vi "Micro-PL v10.6.1.vi"() -> ()   [LabVIEW 2010]
uses:
  drivers/Oxford ITC/ITCAPPS.LLB/ITCSetup.ctl
  drivers/Oxford ITC/ITCSUBS.LLB/ITCIO.ctl
  drivers/Oxford ITC/BUSGEN.LLB/OxfordAddress.ctl
  drivers/Oxford ITC/ITCSUBS.LLB/ITCVersion.ctl
  subvi/NPC3SG/TypeDefs/NPC3SG Live Controls.ctl
  subvi/NPC3SG/TypeDefs/NPC3SG Current Values.ctl
  subvi/NPC3SG/TypeDefs/NPC3SG Set Positions.ctl
  subvi/ITC503/TypeDefs/ITC503 Settings.ctl
  subvi/ITC503/TypeDefs/ITC503 Current Values.ctl
  subvi/iHR550/TypeDefs/iHR Current Values.ctl
  subvi/iHR550/TypeDefs/iHR Settings.ctl
  subvi/Mapping/TypeDefs/Mapping Spectra Params.ctl
  <vilib>/Utility/miscctls.llb/LVBoundsTypeDef.ctl
  subvi/Symphony/TypeDefs/Symphony Area Format.ctl
  <vilib>/Utility/miscctls.llb/LVPointTypeDef.ctl
  subvi/Mapping/TypeDefs/Mapping Input Parameters v10.6.0.ctl
  subvi/Global Variables.vi
  <vilib>/Analysis/NI_AALBase.lvlib
panel:
  out "Spectrum Raw PX":dbl[][](array[numeric])
  out "Image Raw":i32[][](array[numeric])
  in  "Wavelength Recalculate":bool
  out "CCD Error":errorcluster
  out "Firmware":string="V1.20 CCD_4000"
  out "CCD Gain Number":i32[](array[numeric])=[10, 11, 12, 13, 8, 2]
  out "CCD ADC Number":i32[](array[numeric])=[0, 1, 2, 3, 4]
  out "JYCCDLib.IJYCCDReqd":refnum<k7>
  out "Spectrum Raw WL":dbl[][](array[numeric])
  out "Mapping State Storage":bool
  out "Drive Copy Target":bool
  in  "CCD Shutter":bool caption="Shutter:"
  out "Measurement Running":bool
  out "ITC Running":bool
  out "Drive Running":bool
  out "CCD Running":bool
  out "Mono Running":bool
  in  "Exit":bool
  out "Mono Status":bool
  out "Drive Status":bool
  out "CCD Status":bool
  out "ITC Status":bool
  in  "Register":enum32{"Devices", "Acquisition / Mapping"}(tab)
  out "CCD Temp Graph":dbl(graph)=-134.538067
  in  "CCD Gain":u16(ring)=1 caption="Gain Mode" items=["High Light", "Best Dynamic Range", "High Sensitivity"]
  in  "Image Mode":bool caption="Image Mode?"
  in  "CCD Names":u16(ring) caption="CCD ID" items=["Symphony II"]
  in  "CCD Connect":bool
  out "CCD Temperature":dbl caption="Temp. (K)" min=10.0 max=160.0 step=0.1 format="%.1f"
  out "CCD Pixel X":i32=2048 caption="X Pixels"
  out "CCD Pixel Y":i32=512 caption="Y Pixels"
  out "CCD Data Size":i32=2048 caption="Data Size"
  in  "CCD ADC":u16(ring) caption="ADC Frequency" items=["20 kHz       ", " 1 MHz       ", " 1 MHz Ultra ", "500 kHz Wrap"]
  in  "CCD Configure":bool
  in  "CCD Area":T1={"XStart"=1, "YStart"=1, "XStop"=2048, "YStop"=512, "XBin"=1, "YBin"=1}
  in  "Snapshot Folder":path=path "C:/Users/WET-KORR/Desktop/Screenshots"
  in  "Camera Name":string="HD USB Camera"
  out "CCD IDs":u16(ring) items=["CCD1"]
  out "ITC Current Values":T2 {"ITC503 Gradient" format="%.2f"; "ITC503 Setpoint" min=-273.0 max=300000.0 step=0.0001 format="%.1f"; "ITC503 I" format="%_1f"; "ITC503 P" format="%_1f"; "ITC503 Temperature" min=0.0 max=1645.0 step=1e-05 format="%.2f"; "ITC503 Heater" min=0.0 max=100.0 step=0.01 scale=0.0..100.0}
  in  "ITC Settings":T3={"ITC503 Set Setpoint"=0.0, "ITC503 Set Auto Heater"=TRUE, "ITC503 Set Auto PID"=TRUE, "P"=0.0, "I"=0.0, "D"=0.0} {"D" min=0.0 max=100.0 step=0.1 format="%.1f"; "I" min=0.0 max=100.0 step=0.1 format="%.1f"; "P" min=0.0 max=100.0 step=0.1 format="%.1f"; "ITC503 Set Setpoint" min=-273.0 max=300000.0 step=0.1 format="%.1f"}
  in  "ITC Configure":bool
  in  "ITC Connect":bool
  in  "ITC Selector":u16(ring) caption="Select Device" items=["ITC503s"]
  out "Drive Current Values":T4 {"Drive Z Position" min=-273.0 max=300000.0 step=0.0001 format="%.3f"; "Drive Y Position" min=-273.0 max=300000.0 step=0.0001 format="%.3f"; "Drive X Position" min=-273.0 max=300000.0 step=0.0001 format="%.3f"}
  in  "Drive Connection":refnum<visa-resource-name>="COM6" caption="COM Port"
  in  "Drive Connect":bool
  in  "Mono Force Init":bool=TRUE caption="iHR550 Force Init"
  in  "Mono Connect":bool
  in  "Mono ID":string(combo)="iHR550" caption="Monochromator ID"
  out "Mono Timing":u32 caption="Mono"
  out "Drive Timing":u32 caption="Drive"
  out "ITC Timing":u32 caption="ITC"
  out "CCD Timing":u32 caption="CCD"
  in  "Spectrum Axis":u16(ring)=1 caption="Axis" items=["Pixel", "Wavelength", "Energy"]
  in  "Spectrum Autosave":bool caption="iHR550 Force Init"
  in  "CCD Preview":bool
  in  "CCD Acquire":bool
  in  "Spectrum Settings":T5={"Integration Time"=1.0, "Repetitions"=1, "Mapping Spectra"=TRUE} caption="Mapping Spectra Settings" {"Repetitions" min=1 max=100 step=1; "Integration Time" min=0.1 max=6000.0 step=0.1 format="%.1f"}
  in  "CCD Current Rep.":string="0/0"
  out "Spectrum":cluster{dbl[], dbl[]}[](graph)
  in  "Spectrum Noise":i64 caption="Noise Level"
  in  "Spectrum Load":bool
  in  "Spectrum Save":bool
  out "Image":dbl[][](graph)
  in  "Spectrum Maximize":bool
  in  "Video Show":bool
  in  "Drive GoTo":bool caption="Objective Move Abs."
  in  "Drive New Positions":T6 {"Drive X Set" min=10.0 max=160.0 step=0.1 format="%.3f"; "Drive Z Set" min=10.0 max=160.0 step=0.1 format="%.3f"; "Drive Y Set" min=10.0 max=160.0 step=0.1 format="%.3f"}
  out "Drive Live Current Values":T4 {"Drive Z Position" min=-273.0 max=300000.0 step=0.0001 format="%.3f"; "Drive Y Position" min=-273.0 max=300000.0 step=0.0001 format="%.3f"; "Drive X Position" min=-273.0 max=300000.0 step=0.0001 format="%.3f"}
  in  "Drive Live Controls":T7={"Snapshot"=FALSE, "Move Step"=0.5, "Move Home"=FALSE, "Move Down"=FALSE, "Move Up"=FALSE, "Move Left"=FALSE, "Move Right"=FALSE, "Move Out"=FALSE, "Move In"=FALSE} {"Move Step" min=0.0 max=30.0 step=0.1 format="%.3f"}
  in  "Mapping Start":bool
  in  "Mono Configure":bool
  in  "Mono Settings":T8={"iHR550 Set Exit Mirror"=2, "iHR550 Set Side Exit"=0.0, "iHR550 Set Front Entrance"=0.0, "iHR550 Set Wavelength"=897.9988, "iHR550 Set Grating"=0, "iHR550 Set Grating Switch"=FALSE, "iHR550 Set Wavelength Switch"=FALSE, "iHR550 Set Mirror Switch"=FALSE, "iHR550 Set Slits Switch"=FALSE} {"iHR550 Set Grating" items=["1800"=1, "600"=2, "150"=3]; "iHR550 Set Wavelength" min=0.0 max=1500.0 step=1.0; "iHR550 Set Side Exit" min=0.0 max=2000.0 step=1.0; "iHR550 Set Exit Mirror" items=["Front"=2, "Side"=3]}
  out "Mono Current Values":T9={"iHR 550 Front Entrance"=0.0, "iHR550 Side Exit"=0.0, "iHR550 Wavelength"=897.9988, "iHR550 Exit Mirror"=2, "iHR550 Grating"="1", "Grating Index"=1} {"iHR550 Exit Mirror" items=["EntranceMirror", "ExitMirror", "Front", "Side"]}
  out "ITC Temp Storage":dbl
  out "Runtime":u32
  out "ITC Gradient Time":i64
  out "ITC Read":bool
  out "CCD Read":bool
  out "Mono Read":bool
  out "Drive Read":bool
  out "Spectrum Properties":cluster{"Position":T10, "Plot Area Size":T10}={"Position"={"Width"=36, "Height"=367}, "Plot Area Size"={"Width"=496, "Height"=264}}
  in  "Auto Folder":path caption="Ausgewählter Pfad"
  out "Wavelengths (nm)":dbl[](array[numeric])
  out "iHR550 RefNum":refnum<k7> caption="Mono RefNum out"
  out "ITC Setup":T11={"Description"="", "IO Info"={"Address"={"Com Port"=1, "ISOBUS Address"=1, "GPIB Address"=24, "Communication"=enum."ISOBUS"}, "Version"=enum."ITC503", "Ch 1 dec places"=1, "Ch 2 dec places"=1, "Ch 3 dec places"=1, "Ch1 Name"="", "Ch2 Name"="", "Ch3 Name"=""}}
  # "Correlation Setup"
  # "Active"
  # "Active"
  # "ITC"
  # "iHR"
  # "Drive"
  # "CCD"
  # "Status"
  # "CCD"
  # "ITC"
  # "iHR"
  # "Drive"
  # "CCD"
  # "Video"
  # "Cryostat"
  # "Objective Drive"
  # "Monochromator"
  # "Timing"
  # "CCD"
  # "Acquisition"
  # "Drive Control"
  # "XY"
  # "Z"
  # "Mapping"
  # "Launch the Spectral Mapping VI and Raman Tool Set 2.0 in a new window."
  # "Monochromator"
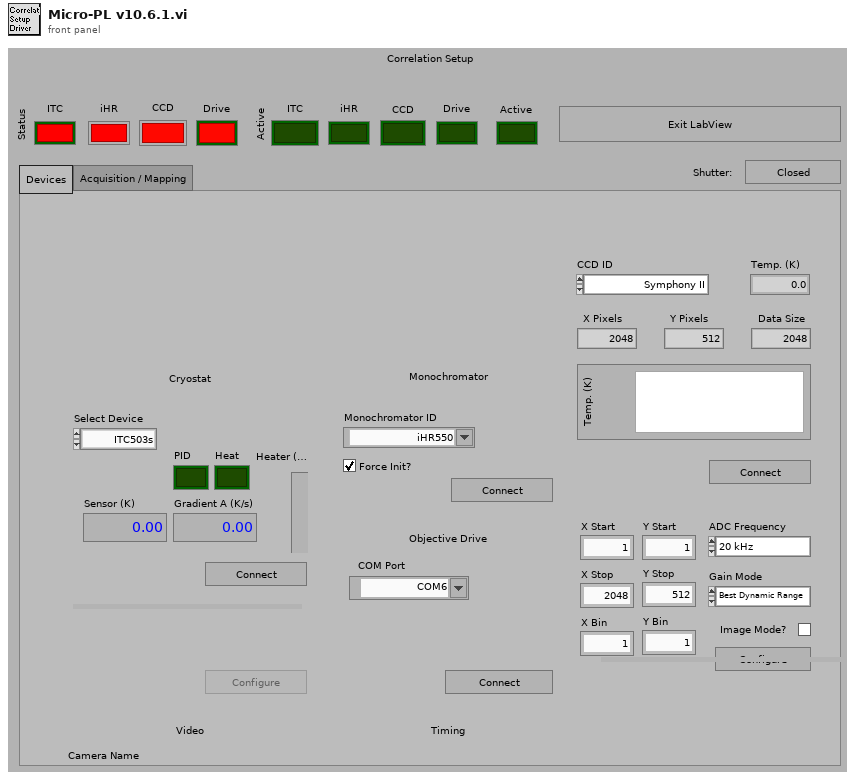
[diagram p1: front panel]
types:
  T1 = typedef "Symphony Area Format.ctl" = cluster{"XStart":i32, "YStart":i32, "XStop":i32, "YStop":i32, "XBin":i32, "YBin":i32}
  T2 = typedef "ITC503 Current Values.ctl" = cluster{"ITC503 Heater":dbl, "ITC503 Temperature":dbl, "ITC503 P":dbl, "ITC503 I":dbl, "ITC503 D":dbl, "ITC503 Setpoint":dbl, "ITC503 Gradient":dbl, "ITC503 Heater Auto":bool, "ITC503 PID Auto":bool}
  T3 = typedef "ITC503 Settings.ctl" = cluster{"ITC503 Set Setpoint":dbl, "ITC503 Set Auto Heater":bool, "ITC503 Set Auto PID":bool, "P":dbl, "I":dbl, "D":dbl}
  T4 = typedef "NPC3SG Current Values.ctl" = cluster{"Drive X Position":dbl, "Drive Y Position":dbl, "Drive Z Position":dbl}
  T5 = typedef "Mapping Spectra Params.ctl" = cluster{"Integration Time":dbl, "Repetitions":u16, "Mapping Spectra":bool}
  T6 = typedef "NPC3SG Set Positions.ctl" = cluster{"Drive X Set":dbl, "Drive Y Set":dbl, "Drive Z Set":dbl}
  T7 = typedef "NPC3SG Live Controls.ctl" = cluster{"Snapshot":bool, "Move Step":dbl, "Move Home":bool, "Move Down":bool, "Move Up":bool, "Move Left":bool, "Move Right":bool, "Move Out":bool, "Move In":bool}
  T8 = typedef "iHR Settings.ctl" = cluster{"iHR550 Set Exit Mirror":u16, "iHR550 Set Side Exit":dbl, "iHR550 Set Front Entrance":dbl, "iHR550 Set Wavelength":dbl, "iHR550 Set Grating":u16, "iHR550 Set Grating Switch":bool, "iHR550 Set Wavelength Switch":bool, "iHR550 Set Mirror Switch":bool, "iHR550 Set Slits Switch":bool}
  T9 = typedef "iHR Current Values.ctl" = cluster{"iHR 550 Front Entrance":dbl, "iHR550 Side Exit":dbl, "iHR550 Wavelength":dbl, "iHR550 Exit Mirror":i32, "iHR550 Grating":string, "Grating Index":i32}
  T10 = typedef "LVBoundsTypeDef.ctl" = cluster{"Width":u32, "Height":u32}
  T11 = typedef "ITCSetup.ctl" = cluster{"Description":string, "IO Info":T12}
  T12 = typedef "ITCIO.ctl" = cluster{"Address":T13, "Version":T14, "Ch 1 dec places":i16, "Ch 2 dec places":i16, "Ch 3 dec places":i16, "Ch1 Name":string, "Ch2 Name":string, "Ch3 Name":string}
  T13 = typedef "OxfordAddress.ctl" = cluster{"Com Port":i32, "ISOBUS Address":i32, "GPIB Address":i16, "Communication":enum16{"RS232", "ISOBUS", "GPIB", "Gateway"}}
  T14 = typedef "ITCVersion.ctl" = enum16{"ITC502", "ITC503", "ITC601"}
  T15 = enum8{"Enabled", "Disabled", "Disabled and Grayed Out"}
  T16 = typedef "LVPointTypeDef.ctl" = cluster{"Horizontal":i16, "Vertical":i16}
  T17 = enum16{"fire", "rainbow", "gray", "inverse gray", "ice", "original"}
  T18 = typedef "Mapping Input Parameters v10.6.0.ctl" = cluster{"Drive Connection Port":refnum<visa-resource-name>, "ITC503 Current Values":T2, "Wavelengths (nm)":dbl[], "Drive Current Values":T4, "iHR Current Values":T9, "Spectra Settings":T5, "CCD3500 Temperature":dbl, "Simulate Drive":bool, "Simulate Spectra":bool, "JYCCDLib.IJYCCDReqd":refnum<k7>, "CCD Area":T1, "CCD Gain":u16, "CCD ADC":u16}
  T19 = cluster{"Intensities":dbl[], "Wavelengths":dbl[]}[]
  T20 = typedef "LVPositionTypeDef.ctl" = cluster{"Left":i32, "Top":i32}
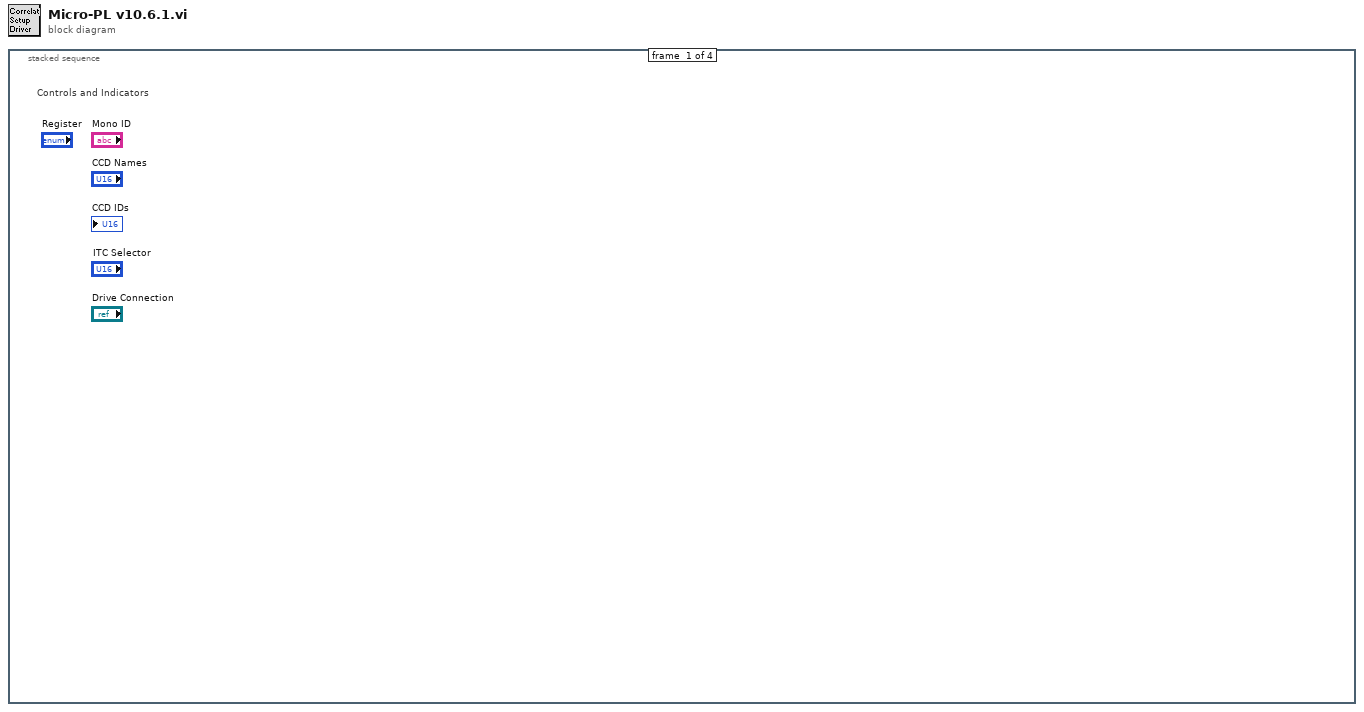
[diagram p0: block diagram]
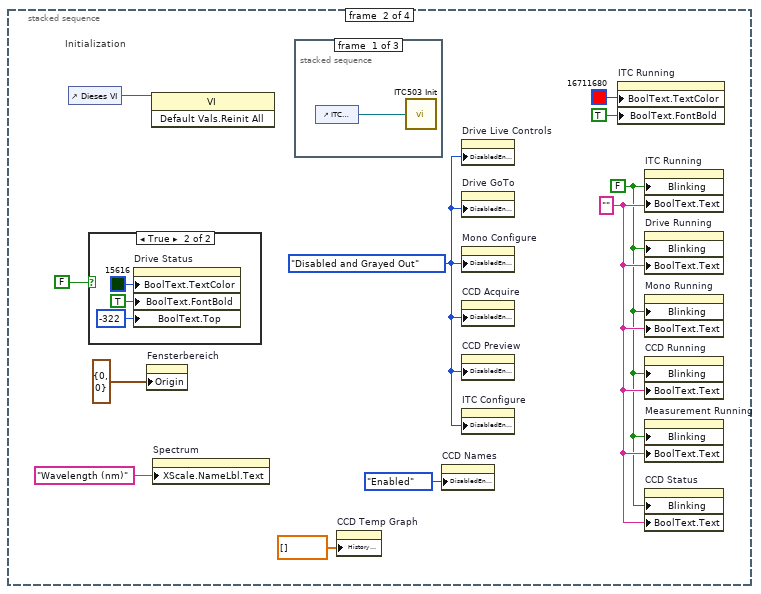
[diagram p2: hidden frame]
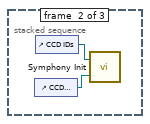
[diagram p3: hidden frame]
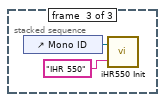
[diagram p4: hidden frame]
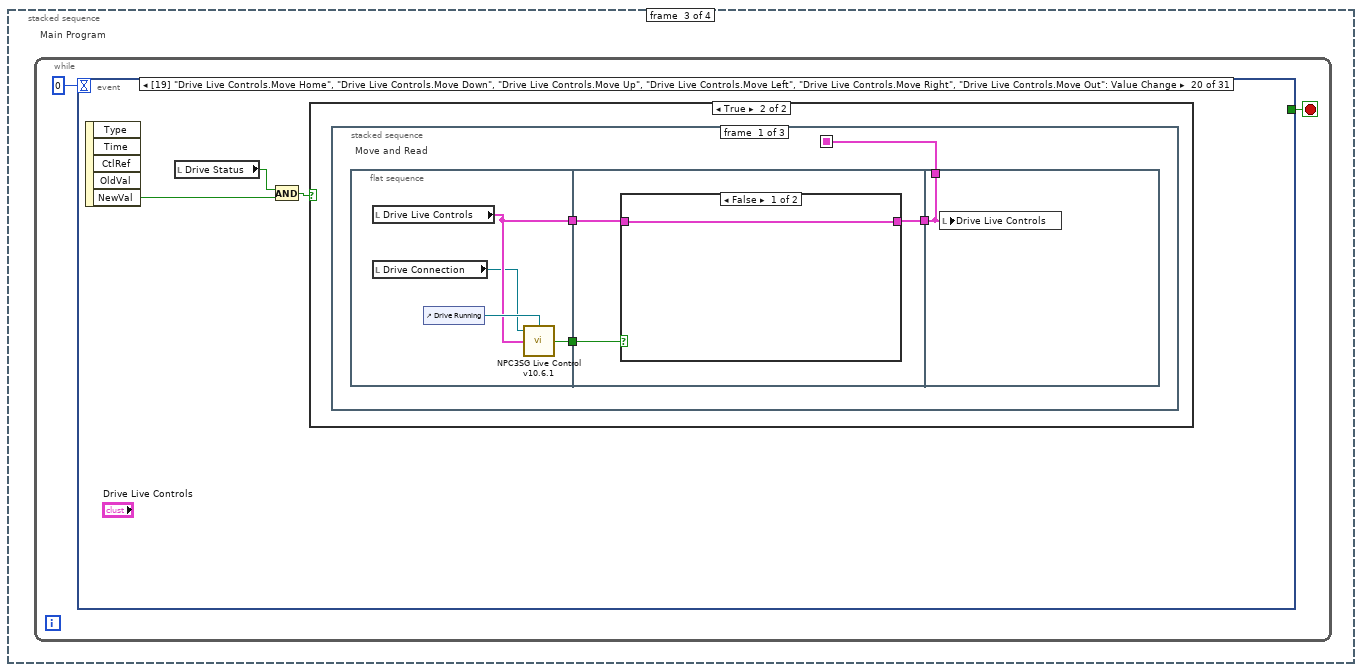
[diagram p6: hidden frame]
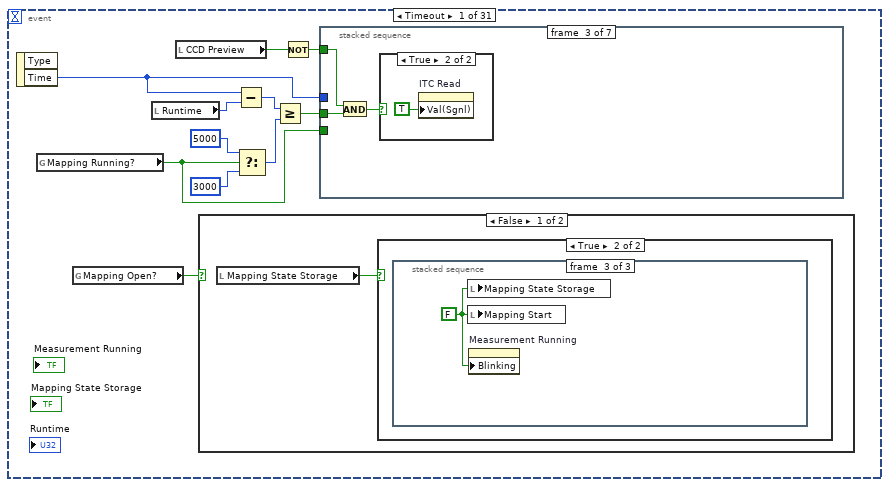
[diagram p7: hidden frame]
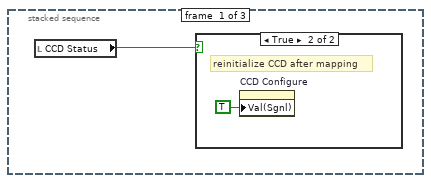
[diagram p9: hidden frame]
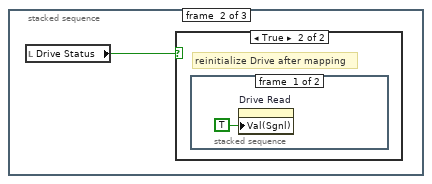
[diagram p11: hidden frame]
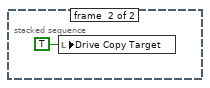
[diagram p13: hidden frame]
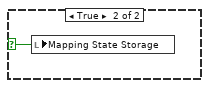
[diagram p14: hidden frame]
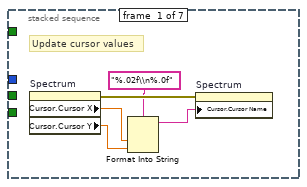
[diagram p15: hidden frame]
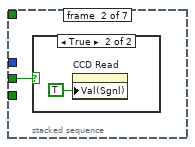
[diagram p16: hidden frame]
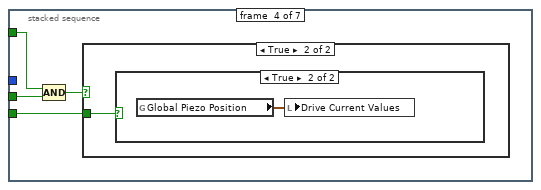
[diagram p19: hidden frame]
diagram:
  n1 = stacked-sequence {
    frame #0 {
      # "Controls and Indicators"
    }
    frame #1 {
      w3 = "" ("Boolean Text.Text")
      w2 = FALSE ("Blinking")
      w8 = T15."Disabled and Grayed Out" ("Deaktiviert")
      # "Initialization"
      n2 = control-ref of="Dieses VI"() -> (w11:refnum<vi>)
      n3 = case shown="True" FALSE {
        frame False {
        }
        frame True {
          n4 = property on="Drive Status" class="Bool (strict)"("BoolText.TextColor"=u32 15616, "BoolText.FontBold"=TRUE ("Boolescher Text.Schriftart:Fett"), "BoolText.Top"=-322 ("Boolescher Text.Position:Oben")) -> ()  [unwired: 2 in, 2 out]
        }
      }
      n5 = property on="Fensterbereich" class="Pane"("Origin"=T16 {"Horizontal"=0, "Vertical"=0}) -> ()  [unwired: 2 in, 2 out]
      n6 = invoke class="VI" method="Default Vals.Reinit All"(reference=w11) -> ()  [unwired: 2 in, 3 out]
      n7 = property on="Spectrum" class="XYGraph (strict)"("XScale.NameLbl.Text"="Wavelength (nm)" ("X Scale.Name Label.Text")) -> ()  [unwired: 2 in, 2 out]
      n8 = stacked-sequence {
        frame #0 {
          n9 = control-ref of="ITC Selector"() -> (w12:refnum<vi>)
          n10 = call "ITC503 Init.vi"("ITC Selector"=w12) -> ()  [unwired: 1 in]
        }
        frame #1 {
          n11 = control-ref of="CCD Names"() -> (w13:refnum<vi>)
          n12 = control-ref of="CCD IDs"() -> (w14:refnum<vi>)
          n13 = call "Symphony Init.vi"("Device Names"=w13, "Device IDs"=w14) -> ()
        }
        frame #2 {
          n14 = control-ref of="Mono ID"() -> (w16:refnum<vi>)
          n15 = call "iHR550 Init.vi"("Mono ID"=w16, "Target ID"="IHR 550") -> ()  [unwired: 1 in]
        }
      }
      n16 = property on="CCD Temp Graph" class="WFChart (strict)"("History Data"=dbl[] []) -> ()  [unwired: 2 in, 2 out]
      n17 = property on="CCD Names" class="Ring (strict)"("DisabledEnum"=T15."Enabled" ("Disabled")) -> ()  [unwired: 2 in, 2 out]
      n18 = property on="Drive Live Controls" class="Clust (strict)"("DisabledEnum"=w8) -> ()  [unwired: 2 in, 2 out]
      n19 = property on="Drive GoTo" class="Bool (strict)"("DisabledEnum"=w8) -> ()  [unwired: 2 in, 2 out]
      n20 = property on="Mono Configure" class="Bool (strict)"("DisabledEnum"=w8) -> ()  [unwired: 2 in, 2 out]
      n21 = property on="CCD Acquire" class="Bool (strict)"("DisabledEnum"=w8) -> ()  [unwired: 2 in, 2 out]
      n22 = property on="CCD Preview" class="Bool (strict)"("DisabledEnum"=w8) -> ()  [unwired: 2 in, 2 out]
      n23 = property on="ITC Configure" class="Bool (strict)"("DisabledEnum"=w8) -> ()  [unwired: 2 in, 2 out]
      n24 = property on="ITC Running" class="Bool (strict)"("BoolText.TextColor"=u32 16711680, "BoolText.FontBold"=TRUE ("Boolean Text.Font:Bold")) -> ()  [unwired: 2 in, 2 out]
      n25 = property on="ITC Running" class="Bool (strict)"("Blinking"=w2, "BoolText.Text"=w3) -> ()  [unwired: 2 in, 2 out]
      n26 = property on="Drive Running" class="Bool (strict)"("Blinking"=w2, "BoolText.Text"=w3) -> ()  [unwired: 2 in, 2 out]
      n27 = property on="Mono Running" class="Bool (strict)"("Blinking"=w2, "BoolText.Text"=w3) -> ()  [unwired: 2 in, 2 out]
      n28 = property on="CCD Running" class="Bool (strict)"("Blinking"=w2, "BoolText.Text"=w3) -> ()  [unwired: 2 in, 2 out]
      n29 = property on="Measurement Running" class="Bool (strict)"("Blinking"=w2, "BoolText.Text"=w3) -> ()  [unwired: 2 in, 2 out]
      n30 = property on="CCD Status" class="Bool (strict)"("Blinking"=w2, "BoolText.Text"=w3) -> ()  [unwired: 2 in, 2 out]
    }
    frame #2 {
      # "Main Program"
      n31 = while "Main-Program" {
        stop <- w21 stop-if-true
        n32 = event shown="[19] \"Drive Live Controls.Move Home\", \"Drive Live Controls.Move Down\", \"Drive Live Controls.Move Up\", \"Drive Live Controls.Move Left\", \"Drive Live Controls.Move Right\", \"Drive Live Controls.Move Out\": Value Change" {
          selector: _ -> [_ _ _ _ _ _ _ _ _ _ _ _ _ _ _ _ _ _ _ _ _ _ _ _ _ _ _ _ _ _ _]
          dyn-events: _ -> [_ _ _ _ _ _ _ _ _ _ _ _ _ _ _ _ _ _ _ _ _ _ _ _ _ _ _ _ _ _ _]
          timeout: 0 -> [_ _ _ _ _ _ _ _ _ _ _ _ _ _ _ _ _ _ _ _ _ _ _ _ _ _ _ _ _ _ _]
          tunnel: [_ w70 _ _ _ _ _ _ _ _ _ _ _ _ _ _ _ _ _ _ _ _ _ _ _ _ _ _ _ _ _] -> w21
          event Timeout {
            n33 = event-data() -> ("Time"=w28:u32)  [unwired: 1 in, 1 out]
            n34 = global read "Global Variables.vi" "Mapping Running?"() -> (w23:bool)
            n35 = global read "Global Variables.vi" "Mapping Open?"() -> (w22:bool)
            n36 = local read "Runtime"() -> (w27:u32)
            n37 = local read "CCD Preview"() -> (w30:bool)
            n38 = case shown="False" w22 {
              selector: w22 -> [_ w40]
              frame False {
                n39 = local read "Mapping State Storage"() -> (w33:bool)
                n40 = case shown="True" w33 {
                  frame False {
                  }
                  frame True {
                    n41 = stacked-sequence {
                      frame #0 {
                        n42 = local read "CCD Status"() -> (w34:bool)
                        n43 = case shown="True" w34 {
                          frame False {
                          }
                          frame True {
                            # "reinitialize CCD after mapping"
                            n44 = property on="CCD Configure" class="Bool (strict)"("Val(Sgnl)"=TRUE ("Value (Signaling)")) -> ()  [unwired: 2 in, 2 out]
                          }
                        }
                      }
                      frame #1 {
                        n45 = local read "Drive Status"() -> (w36:bool)
                        n46 = case shown="True" w36 {
                          frame False {
                          }
                          frame True {
                            # "reinitialize Drive after mapping"
                            n47 = stacked-sequence {
                              frame #0 {
                                n48 = property on="Drive Read" class="Bool (strict)"("Val(Sgnl)"=TRUE ("Value (Signaling)")) -> ()  [unwired: 2 in, 2 out]
                              }
                              frame #1 {
                                n49 = local write "Drive Copy Target"(TRUE ("Copy Drive Target")) -> ()
                              }
                            }
                          }
                        }
                      }
                      frame #2 {
                        w39 = FALSE ("Mapping Start")
                        n50 = local write "Mapping State Storage"(w39) -> ()
                        n51 = local write "Mapping Start"(w39) -> ()
                        n52 = property on="Measurement Running" class="Bool (strict)"("Blinking"=w39) -> ()  [unwired: 2 in, 2 out]
                      }
                    }
                  }
                }
              }
              frame True {
                n53 = local write "Mapping State Storage"(w40) -> ()
              }
            }
            n54 = Subtract(x=w28, y=w27) -> (x-y=w31:u32)
            n55 = Select(t=u32 5000 ("y"), s=w23, f=u32 3000 ("y")) -> (s? t:f=w24:u32)
            n56 = Greater Or Equal?(x=w31, y=w24) -> (x >= y?=w32:bool)
            n57 = Not(x=w30) -> (.not. x?=w29:bool)
            n58 = stacked-sequence {
              tunnel: w32 -> [_ w46 w50 w55 w62 _ w67]
              tunnel: w28 -> [_ _ _ _ _ _ w68]
              tunnel: w29 -> [_ _ w49 w54 w61 w64 _]
              tunnel: w23 -> [_ _ _ w52 w59 _ _]
              frame #0 {
                # "Update cursor values"
                n59 = property on="Spectrum" class="XYGraph (strict)"() -> (error out=w45:errorcluster, "Cursor.Cursor X"=w44:dbl, "Cursor.Cursor Y"=w43:dbl)  [unwired: 2 in, 1 out]
                n60 = Format Into String(format string="%.02f\\n%.0f", w44, w43) -> (resulting string=w41:string)  [unwired: 2 in, 1 out]
                n61 = property on="Spectrum" class="XYGraph (strict)"(error in=w45, "Cursor.Cursor Name"=w41) -> ()  [unwired: 1 in, 2 out]
              }
              frame #1 {
                n62 = case shown="True" w46 {
                  frame False {
                  }
                  frame True {
                    n63 = property on="CCD Read" class="Bool (strict)"("Val(Sgnl)"=TRUE ("Value (Signaling)")) -> ()  [unwired: 2 in, 2 out]
                  }
                }
              }
              frame #2 {
                n64 = And(x=w49, y=w50) -> (x .and. y?=w48:bool)
                n65 = case shown="True" w48 {
                  frame False {
                  }
                  frame True {
                    n66 = property on="ITC Read" class="Bool (strict)"("Val(Sgnl)"=TRUE ("Value (Signaling)")) -> ()  [unwired: 2 in, 2 out]
                  }
                }
              }
              frame #3 {
                n67 = Compound Arithmetic op=AND(w54, w55) -> (w53:bool)
                n68 = case shown="True" w53 {
                  tunnel: w52 -> [_ w56]
                  frame False {
                  }
                  frame True {
                    n69 = case shown="True" w56 {
                      frame False {
                        n70 = property on="Drive Read" class="Bool (strict)"("Val(Sgnl)"=TRUE ("Value (Signaling)")) -> ()  [unwired: 2 in, 2 out]
                      }
                      frame True {
                        n71 = global read "Global Variables.vi" "Global Piezo Position"() -> (w58:T4)
                        n72 = local write "Drive Current Values"(w58) -> ()
                      }
                    }
                  }
                }
              }
              frame #4 {
                n73 = Compound Arithmetic op=AND(w61, w62, w59) -> (w60:bool)
                n74 = case shown="True" w60 {
                  frame False {
                  }
                  frame True {
                    n75 = property on="Mono Read" class="Bool (strict)"("Val(Sgnl)"=TRUE ("Value (Signaling)")) -> ()  [unwired: 2 in, 2 out]
                  }
                }
              }
              frame #5 {
                n76 = case shown="False" w64 {
                  frame False {
                    n77 = flat-sequence {
                      frame #0 {
                        w65 = u32 50  # CCD buffer
                        n78 = Wait (ms)(milliseconds to wait=w65) -> ()  [unwired: 1 out]
                      }
                      frame #1 {
                        n79 = property on="CCD Acquire" class="Bool (strict)"("Val(Sgnl)"=TRUE ("Wert (signalisierend)")) -> ()  [unwired: 2 in, 2 out]
                      }
                    }
                  }
                  frame True {
                  }
                }
              }
              frame #6 {
                # "Set runtime counter"
                n80 = case shown="True" w67 {
                  tunnel: w68 -> [_ w69]
                  frame False {
                  }
                  frame True {
                    n81 = local write "Runtime"(w69) -> ()
                  }
                }
              }
            }
          }
          event "Exit": Value Change {
            n82 = event-data() -> ("NewVal"=w70:bool)  [unwired: 1 in, 4 out]
            n83 = stacked-sequence {
              frame #0 {
                n84 = local read "CCD Status"() -> (w71:bool)
                n85 = case shown="True" w71 {
                  frame False {
                  }
                  frame True {
                    n86 = local read "JYCCDLib.IJYCCDReqd"() -> (w72:refnum<k7>)
                    n87 = Close Reference(reference=w72) -> ()  [unwired: 1 in, 1 out]
                  }
                }
              }
              frame #1 {
                n88 = local read "Drive Status"() -> (w73:bool)
                n89 = case shown="True" w73 {
                  frame False {
                  }
                  frame True {
                    n90 = local read "Drive Connection"() -> (w74:refnum<visa-resource-name>)
                    n91 = call "NPC3SG Close.vi"("Drive Visa Name"=w74) -> ()  [unwired: 4 in]
                  }
                }
              }
            }
          }
          event "Mono Connect": Value Change {
            n92 = event-data() -> ("NewVal"=w75:bool)  [unwired: 1 in, 4 out]
            n93 = stacked-sequence {
              tunnel: w75 -> [_ w78 _]
              frame #0 {
                n94 = property on="Mono Running" class="Bool (strict)"("Blinking"=TRUE ("Blinkend")) -> ()  [unwired: 2 in, 2 out]
              }
              frame #1 {
                n95 = case shown="False" w78 {
                  selector: w78 -> [w82 _]
                  tunnel: [w82 w94] -> w77
                  frame False {
                    # "disconnect"
                  }
                  frame True {
                    # "connect"
                    n96 = local read "Mono Force Init"() -> (w92:bool)
                    n97 = control-ref of="iHR550 Set Grating"() -> (w93:refnum<vi>)
                    n98 = local read "Mono ID"() -> (w95:string)
                    n99 = call "iHR550 Connect.vi"("Force\nInitialization"=w92, "Grating Selector"=w93, "Mono ID"=w95) -> ("Initialized"=w94:bool, "iHR550 RefNum"=w91:refnum<k7>)  [unwired: 2 in, 4 out]
                    n100 = local write "iHR550 RefNum"(w91) -> ()
                    n101 = call "iHR550 Read Values v10.5.0.vi"("JYMONOLib.IJYMonoReqd"=w91) -> ("iHR Current Values"=w83:T9)  [unwired: 1 in]
                    n102 = Unbundle By Name(w83) -> ("iHR 550 Front Entrance"=w89:dbl, "iHR550 Side Exit"=w88:dbl, "iHR550 Wavelength"=w87:dbl, "iHR550 Exit Mirror"=w86:i32, "Grating Index"=w84:i32)
                    n103 = local write "Mono Current Values"(w83) -> ()
                    n104 = Bundle By Name(cluster=T8 {"iHR550 Set Exit Mirror"=0, "iHR550 Set Side Exit"=0.0, "iHR550 Set Front Entrance"=0.0, "iHR550 Set Wavelength"=0.0, "iHR550 Set Grating"=0, "iHR550 Set Grating Switch"=FALSE, "iHR550 Set Wavelength Switch"=FALSE, "iHR550 Set Mirror Switch"=FALSE, "iHR550 Set Slits Switch"=FALSE} ("iHR Settings"), "iHR550 Set Front Entrance"=w89, "iHR550 Set Side Exit"=w88, "iHR550 Set Wavelength"=w87, "iHR550 Set Exit Mirror"=w86, "iHR550 Set Grating"=w84) -> (w85:T8)
                    n105 = local write "Mono Settings"(w85) -> ()
                  }
                }
                n106 = case shown="False" w77 {
                  tunnel: [T15."Disabled and Grayed Out" ("Deaktiviert") T15."Enabled" ("Deaktiviert")] -> w79
                  frame False {
                  }
                  frame True {
                  }
                }
                n107 = local write "Mono Connect"(w77) -> ()
                n108 = local write "Mono Status"(w77) -> ()
                n109 = property on="Mono Configure" class="Bool (strict)"("DisabledEnum"=w79) -> ()  [unwired: 2 in, 2 out]
              }
              frame #2 {
                w97 = TRUE ("Wert (signalisierend)")
                w96 = FALSE ("Blinkend")
                n110 = local write "Mono Force Init"(w96) -> ()
                n111 = property on="Mono Running" class="Bool (strict)"("Blinking"=w96) -> ()  [unwired: 2 in, 2 out]
                n112 = property on="Mono Read" class="Bool (strict)"("Val(Sgnl)"=w97) -> ()  [unwired: 2 in, 2 out]
                n113 = property on="Wavelength Recalculate" class="Bool (strict)"("Val(Sgnl)"=w97) -> ()  [unwired: 2 in, 2 out]
              }
            }
          }
          event "Mono Read": Value Change {
            n114 = event-data() -> ("NewVal"=w101:bool)  [unwired: 1 in, 4 out]
            n115 = local read "Mono Status"() -> (w100:bool)
            n116 = And(x=w100, y=w101) -> (x .and. y?=w99:bool)
            n117 = case shown="False" w99 {
              tunnel: [u32 0 w103] -> w98
              frame False {
              }
              frame True {
                n118 = stacked-sequence {
                  seq-local: [w104 _ _] -> [_ _ w107]
                  tunnel: [_ _ w108] -> w103
                  frame #0 {
                    n119 = Tick Count (ms)() -> (millisecond timer value=w104:u32)
                  }
                  frame #1 {
                    n120 = local read "iHR550 RefNum"() -> (w106:refnum<k7>)
                    n121 = call "iHR550 Read Values v10.5.0.vi"("JYMONOLib.IJYMonoReqd"=w106) -> ("iHR Current Values"=w105:T9)  [unwired: 1 in]
                    n122 = local write "Mono Current Values"(w105) -> ()
                    n123 = global write "Global Variables.vi" "Global iHR Values"(w105) -> ()
                  }
                  frame #2 {
                    n124 = Tick Count (ms)() -> (millisecond timer value=w109:u32)
                    n125 = Subtract(x=w109, y=w107) -> (x-y=w108:u32)
                  }
                }
              }
            }
            "Mono Timing" <- w98
          }
          event "Mono Configure": Value Change {
            n126 = event-data() -> ("NewVal"=w110:bool)  [unwired: 1 in, 4 out]
            n127 = stacked-sequence {
              tunnel: w110 -> [_ w112 _]
              frame #0 {
                n128 = property on="Mono Running" class="Bool (strict)"("Blinking"=TRUE ("Blinkend")) -> ()  [unwired: 2 in, 2 out]
              }
              frame #1 {
                n129 = local read "Mono Status"() -> (w114:bool)
                n130 = And(x=w114, y=w112) -> (x .and. y?=w113:bool)
                n131 = case shown="True" w113 {
                  frame False {
                  }
                  frame True {
                    n132 = stacked-sequence {
                      frame #0 {
                        w118 = u16 2 items=["Front"=2, "Side"=3] ("Entrance Mirror")
                        n133 = local read "iHR550 RefNum"() -> (w115:refnum<k7>)
                        n134 = local read "Mono Settings"() -> (w116:T8)
                        n135 = call "iHR550 Set Values v10.5.0.vi"("Refnum out"=w115, "Entrance Mirror"=w118, "Target\nSide Entrance"=0.0 ("Target\nSide Entrance"), "iHR Settings"=w116) -> ()  [unwired: 11 in, 1 out]
                      }
                      frame #1 {
                        n136 = property on="Mono Read" class="Bool (strict)"("Val(Sgnl)"=TRUE ("Value (Signaling)")) -> ()  [unwired: 2 in, 2 out]
                      }
                      frame #2 {
                        n137 = property on="Wavelength Recalculate" class="Bool (strict)"("Val(Sgnl)"=TRUE ("Value (Signaling)")) -> ()  [unwired: 2 in, 2 out]
                      }
                    }
                  }
                }
              }
              frame #2 {
                w122 = FALSE ("Blinkend")
                n138 = property on="Mono Read" class="Bool (strict)"("Val(Sgnl)"=TRUE ("Wert (signalisierend)")) -> ()  [unwired: 2 in, 2 out]
                n139 = property on="Mono Running" class="Bool (strict)"("Blinking"=w122) -> ()  [unwired: 2 in, 2 out]
                n140 = local write "Mono Configure"(w122) -> ()
              }
            }
          }
          event "CCD Connect": Value Change {
            n141 = event-data() -> ("NewVal"=w123:bool)  [unwired: 1 in, 4 out]
            n142 = stacked-sequence {
              tunnel: w123 -> [_ w127 _]
              frame #0 {
                n143 = local read "CCD Names"() -> (w124:u16)
                n144 = property on="CCD Running" class="Bool (strict)"("Blinking"=TRUE ("Blinkend")) -> ()  [unwired: 2 in, 2 out]
                n145 = local write "CCD IDs"(w124) -> ()
              }
              frame #1 {
                n146 = case shown="False" w127 {
                  selector: w127 -> [w138 _]
                  tunnel: [w138 w147] -> w129
                  frame False {
                    # "disconnect"
                    n147 = local read "JYCCDLib.IJYCCDReqd"() -> (w137:refnum<k7>)
                    n148 = property on="CCD Status" class="Bool (strict)"("Blinking"=FALSE, "BoolText.Text"="" ("Boolean Text.Text")) -> ()  [unwired: 2 in, 2 out]
                    n149 = local read "CCD Error"() -> (w136:errorcluster)
                    n150 = Close Reference(reference=w137, error in (no error)=w136) -> ()  [unwired: 1 out]
                  }
                  frame True {
                    # "connect"
                    n151 = local read "CCD IDs"() -> (w152:u16)
                    n152 = property on="CCD IDs" class="Ring (strict)"() -> ("Chaînes []"=w151:string[])  [unwired: 2 in, 2 out]
                    n153 = Index Array(array=w151, index=w152) -> (element=w153:string)
                    n154 = call "Initialize CCD.vi"("Unique id:"=w153) -> ("activeYPixels"=w140:i32, "JYCCDLib.IJYCCDReqd"=w154:refnum<k7>, "activeXPixels"=w142:i32, "sortie d'erreur"=w155:errorcluster, "FirmwareVersion"=→"Firmware":string)  [unwired: 3 out]
                    "CCD Pixel X" <- w142
                    "CCD Pixel Y" <- w140
                    n155 = call "Trigger - Disable.vi"("Error In"=w155, "JYCCDLib.IJYCCDReqd"=w154) -> ("Error Out"=w149:errorcluster, "JYCCDLib.IJYCCDReqd"=w160:refnum<k7>)  [unwired: 4 out]
                    n156 = local read "CCD Area"() -> (w146:T1)
                    n157 = Bundle By Name(cluster=w146, "XStart"=1, "XStop"=w142, "YStart"=1, "YStop"=w140, "XBin"=1, "YBin"=1) -> (w145:T1)
                    n158 = local write "CCD Error"(w149) -> ()
                    n159 = call "Init ADC & Gain.vi"("JYCCDLib.IJYCCDReqd"=w160, "input error"=w149) -> ("ADC Number"=w156:i32[], "ADC description"=w158:string[], "Gain Number"=w157:i32[], "Gain description"=w159:string[])
                    n160 = local write "JYCCDLib.IJYCCDReqd"(w160) -> ()
                    n161 = local write "CCD Area"(w145) -> ()
                    n162 = local write "CCD ADC Number"(w156) -> ()
                    n163 = local write "CCD Gain Number"(w157) -> ()
                    n164 = property on="CCD ADC" class="Ring (strict)"("Chaînes []"=w158) -> ()  [unwired: 2 in, 2 out]
                    n165 = property on="CCD Gain" class="Ring (strict)"("Chaînes []"=w159) -> ()  [unwired: 2 in, 2 out]
                    n166 = call <vilib>:"Simple Error Handler.vi"("error in (no error)"=w149) -> ("error?"=w148:bool)  [unwired: 4 in, 4 out]
                    n167 = Not(x=w148) -> (.not. x?=w147:bool)
                  }
                }
                n168 = case shown="False" w129 {
                  tunnel: [T15."Disabled and Grayed Out" ("Deaktiviert") T15."Enabled" ("Deaktiviert")] -> w128
                  tunnel: [T15."Enabled" ("Deaktiviert") T15."Disabled and Grayed Out" ("Deaktiviert")] -> w126
                  frame False {
                  }
                  frame True {
                  }
                }
                n169 = property on="CCD Status" class="Bool (strict)"("BoolText.Visible"=w129) -> ()  [unwired: 2 in, 2 out]
                n170 = local write "CCD Connect"(w129) -> ()
                n171 = local write "CCD Status"(w129) -> ()
                n172 = property on="CCD Acquire" class="Bool (strict)"("DisabledEnum"=w128) -> ()  [unwired: 2 in, 2 out]
                n173 = property on="CCD Preview" class="Bool (strict)"("DisabledEnum"=w128) -> ()  [unwired: 2 in, 2 out]
                n174 = property on="CCD Names" class="Ring (strict)"("Désactivé"=w126) -> ()  [unwired: 2 in, 2 out]
                n175 = property on="CCD IDs" class="Ring (strict)"("Désactivé"=w126) -> ()  [unwired: 2 in, 2 out]
              }
              frame #2 {
                w161 = TRUE ("Wert (signalisierend)")
                n176 = property on="CCD Configure" class="Bool (strict)"("Val(Sgnl)"=w161) -> (error out=w162:errorcluster)  [unwired: 2 in, 1 out]
                n177 = property on="CCD Running" class="Bool (strict)"("Blinking"=FALSE ("Blinkend")) -> ()  [unwired: 2 in, 2 out]
                n178 = property on="CCD Read" class="Bool (strict)"(error in=w162, "Val(Sgnl)"=w161) -> ()  [unwired: 1 in, 2 out]
              }
            }
          }
          event "CCD Read": Value Change {
            n179 = event-data() -> ("NewVal"=w167:bool)  [unwired: 1 in, 4 out]
            n180 = local read "CCD Status"() -> (w166:bool)
            n181 = And(x=w166, y=w167) -> (x .and. y?=w165:bool)
            n182 = case shown="True" w165 {
              tunnel: [u32 0 w169] -> w164
              frame False {
              }
              frame True {
                n183 = stacked-sequence {
                  seq-local: [_ w171 _ _] -> [_ _ w179 _]
                  seq-local: [w170 _ _ _] -> [_ _ _ w190]
                  tunnel: [_ _ _ w191] -> w169
                  frame #0 {
                    n184 = Tick Count (ms)() -> (millisecond timer value=w170:u32)
                  }
                  frame #1 {
                    w172 = u16 1 items=["° Celsius", "Kelvin", "° Farenheit"] ("units")
                    n185 = local read "JYCCDLib.IJYCCDReqd"() -> (w175:refnum<k7>)
                    n186 = local read "CCD Error"() -> (w173:errorcluster)
                    n187 = call "read temperature.vi"("entrée d'erreur (pas d'erreur)"=w173, "units"=w172, "JYCCDLib.IJYCCDReqd"=w175) -> ("error out"=w174:errorcluster, "Current Temperature"=w171:dbl)
                    n188 = local write "CCD Temp Graph"(w171) -> ()
                    n189 = local write "CCD Error"(w174) -> ()
                    n190 = local write "CCD Temperature"(w171) -> ()
                  }
                  frame #2 {
                    n191 = Subtract(x=w179, y=140.0) -> (x-y=w176:dbl)
                    n192 = Absolute Value(x=w176) -> (abs(x)=w177:dbl)
                    n193 = Greater?(x=w177, y=1.0) -> (0:w181:bool)
                    n194 = case shown="False" w181 {
                      selector: w181 -> [w187 w189]
                      tunnel: [cluster{u32, u32}[] [{16713728, 16713728}, {6618880, 6618880}] ("Farben [4]") cluster{u32, u32}[] [{16713728, 16713728}] ("Farben [4]")] -> w182
                      tunnel: [w187 w189] -> w184
                      frame False {
                      }
                      frame True {
                      }
                    }
                    n195 = Number To Fractional String(number=w179, precision (6)=i16 1 ("Genauigkeit (6)")) -> (F-format string=w183:string)  [unwired: 2 in]
                    n196 = global write "Global Variables.vi" "Global CCD Temperature (C)"(w179) -> ()
                    n197 = property on="CCD Status" class="Bool (strict)"("Blinking"=w184, "BoolText.Text"=w183, "Colors [4]"=w182) -> ()  [unwired: 2 in, 2 out]
                  }
                  frame #3 {
                    n198 = Tick Count (ms)() -> (millisecond timer value=w192:u32)
                    n199 = Subtract(x=w192, y=w190) -> (x-y=w191:u32)
                  }
                }
              }
            }
            "CCD Timing" <- w164
          }
          event "CCD Configure": Value Change {
            n200 = event-data() -> ("NewVal"=w194:bool)  [unwired: 1 in, 4 out]
            n201 = local read "CCD Status"() -> (w195:bool)
            n202 = And(x=w195, y=w194) -> (x .and. y?=w193:bool)
            n203 = case shown="True" w193 {
              frame False {
              }
              frame True {
                n204 = stacked-sequence {
                  frame #0 {
                    n205 = local read "Spectrum Settings"() -> (w200:T5)
                    n206 = local read "CCD Gain Number"() -> (w209:i32[])
                    n207 = local read "CCD ADC Number"() -> (w207:i32[])
                    n208 = local read "JYCCDLib.IJYCCDReqd"() -> (w198:refnum<k7>)
                    n209 = local read "CCD ADC"() -> (w206:u16)
                    n210 = local read "CCD Gain"() -> (w208:u16)
                    n211 = Unbundle By Name(w200) -> ("Integration Time"=w199:dbl)
                    n212 = local read "Image Mode"() -> (w203:bool)
                    n213 = local read "CCD Error"() -> (w202:errorcluster)
                    n214 = local read "CCD Area"() -> (w197:T1)
                    n215 = Index Array(array=w207, index=w206) -> (element=w205:i32)
                    n216 = Index Array(array=w209, index=w208) -> (element=w204:i32)
                    n217 = call "Symphony Setup.vi"("JYCCDLib.IJYCCDReqd"=w198, "ADC"=w205, "Image Mode"=w203, "Integration (s)"=w199, "Symphony Area Format"=w197, "Error Input"=w202, "Gain"=w204) -> ("DataSize"=w196:i32, "Error Output"=w201:errorcluster)  [unwired: 7 in]
                    n218 = local write "CCD Error"(w201) -> ()
                    n219 = local write "CCD Data Size"(w196) -> ()
                  }
                  frame #1 {
                    n220 = property on="Wavelength Recalculate" class="Bool (strict)"("Val(Sgnl)"=TRUE ("Value (Signaling)")) -> ()  [unwired: 2 in, 2 out]
                    n221 = local write "CCD Configure"(FALSE ("CCD Configure")) -> ()
                    n222 = local read "Image Mode"() -> (w213:bool)
                    n223 = call "Image Intensity Color Tables.vi"("Map Selector"=T17."original") -> ("Color Map Array"=w211:u32[])  [unwired: 10 in]
                    n224 = Not(x=w213) -> (.not. x?=w212:bool)
                    n225 = property on="Image" class="IntGraph (strict)"("Visible"=w213, "Color Table"=w211) -> ()  [unwired: 2 in, 2 out]
                    n226 = property on="Spectrum" class="XYGraph (strict)"("Visible"=w212) -> ()  [unwired: 2 in, 2 out]
                    n227 = property on="Spectrum Load" class="Bool (strict)"("Visible"=w212) -> ()  [unwired: 2 in, 2 out]
                    n228 = property on="Spectrum Noise" class="DigNum (strict)"("Visible"=w212) -> ()  [unwired: 2 in, 2 out]
                    n229 = property on="CCD Current Rep." class="Str"("Visible"=w212) -> ()  [unwired: 2 in, 2 out]
                  }
                }
              }
            }
          }
          event Value Change {
            n230 = event-data() -> ()  [unwired: 1 in, 5 out]
            n231 = stacked-sequence {
              frame #0 {
                w229 = 1 ("y")
                n232 = local read "CCD Area"() -> (w227:T1)
                n233 = Unbundle By Name(w227) -> ("XBin"=w223:i32, "YBin"=w228:i32)
                n234 = Logarithm Base 2(1:w228) -> (0:w224:dbl)
                n235 = Logarithm Base 2(1:w223) -> (0:w220:dbl)
                n236 = Quotient & Remainder(x=w224, y=w229) -> (x-y*floor(x/y)=w225:dbl, floor(x/y)=w226:dbl)
                n237 = Quotient & Remainder(x=w220, y=w229) -> (x-y*floor(x/y)=w221:dbl, floor(x/y)=w222:dbl)
                n238 = Not Equal To 0?(x=w225) -> (x != 0?=w219:bool)
                n239 = Not Equal To 0?(x=w221) -> (x != 0?=w218:bool)
                n240 = Or(x=w218, y=w219) -> (x .or. y?=w217:bool)
                n241 = case shown="True" w219 {
                  tunnel: w226 -> [_ w234]
                  tunnel: w227 -> [_ w232]
                  frame False {
                  }
                  frame True {
                    n242 = Power Of 2(x=w234) -> (2^x=w233:dbl)
                    n243 = Bundle By Name(cluster=w232, "YBin"=w233) -> (w231:T1)
                    n244 = local write "CCD Area"(w231) -> ()
                  }
                }
                n245 = case shown="True" w218 {
                  tunnel: w222 -> [_ w238]
                  tunnel: w227 -> [_ w236]
                  frame False {
                  }
                  frame True {
                    n246 = Power Of 2(x=w238) -> (2^x=w237:dbl)
                    n247 = Bundle By Name(cluster=w236, "XBin"=w237) -> (w235:T1)
                    n248 = local write "CCD Area"(w235) -> ()
                  }
                }
                n249 = case shown="True" w217 {
                  tunnel: "Binning factor has been adjusted  (must be an exponent of 2)." ("message") -> [_ w230]
                  frame False {
                  }
                  frame True {
                    n250 = One Button Dialog(message=w230) -> ()  [unwired: 1 in, 1 out]
                  }
                }
              }
              frame #1 {
                w257 = "Could not adjust CCD area to fit binning size!" ("message")
                w258 = "CCD area has been adjusted to fit binning size." ("message")
                n251 = local read "CCD Area"() -> (w239:T1)
                n252 = Unbundle By Name(w239) -> ("XStop"=w246:i32, "XStart"=w247:i32, "XBin"=w244:i32)
                n253 = Unbundle By Name(w239) -> ("YStop"=w251:i32, "YStart"=w252:i32, "YBin"=w256:i32)
                n254 = Subtract(x=w246, y=w247) -> (x-y=w240:i32)
                n255 = Subtract(x=w251, y=w252) -> (x-y=w249:i32)
                n256 = Increment(x=w240) -> (x+1=w245:i32)
                n257 = Increment(x=w249) -> (x+1=w253:i32)
                n258 = Quotient & Remainder(x=w245, y=w244) -> (x-y*floor(x/y)=w241:i32, floor(x/y)=w243:i32)
                n259 = Quotient & Remainder(x=w253, y=w256) -> (x-y*floor(x/y)=w250:i32, floor(x/y)=w255:i32)
                n260 = Not Equal To 0?(x=w241) -> (x != 0?=w242:bool)
                n261 = Not Equal To 0?(x=w250) -> (x != 0?=w254:bool)
                n262 = case shown="True" w254 {
                  tunnel: w251 -> [_ w276]
                  tunnel: w252 -> [_ w275]
                  tunnel: w253 -> [_ w274]
                  tunnel: w255 -> [_ w273]
                  tunnel: w256 -> [_ w272]
                  tunnel: w257 -> [_ w266]
                  tunnel: w258 -> [_ w267]
                  tunnel: w239 -> [_ w271]
                  tunnel: ["" ("message") w268] -> w260
                  frame False {
                  }
                  frame True {
                    n263 = Multiply(x=w273, y=w272) -> (x*y=w278:i32)
                    n264 = Subtract(x=w274, y=w278) -> (x-y=w277:i32)
                    n265 = Add(x=w275, y=w277) -> (x+y=w270:i32)
                    n266 = Greater?(x=w276, y=w270) -> (0:w269:bool)
                    n267 = case shown="True" w269 {
                      tunnel: w271 -> [_ w283]
                      tunnel: w270 -> [_ w282]
                      tunnel: [w279 w280] -> w268
                      tunnel: w267 -> [_ w280]
                      tunnel: w266 -> [w279 _]
                      frame False {
                      }
                      frame True {
                        n268 = Bundle By Name(cluster=w283, "YStart"=w282) -> (w281:T1)
                        n269 = local write "CCD Area"(w281) -> ()
                      }
                    }
                  }
                }
                n270 = case shown="True" w242 {
                  tunnel: w243 -> [_ w298]
                  tunnel: w244 -> [_ w297]
                  tunnel: w245 -> [_ w291]
                  tunnel: w246 -> [_ w294]
                  tunnel: w247 -> [_ w292]
                  tunnel: w239 -> [_ w290]
                  tunnel: ["" ("message") w288] -> w261
                  tunnel: w258 -> [_ w287]
                  tunnel: w257 -> [_ w286]
                  frame False {
                  }
                  frame True {
                    n271 = Multiply(x=w298, y=w297) -> (x*y=w296:i32)
                    n272 = Subtract(x=w291, y=w296) -> (x-y=w293:i32)
                    n273 = Add(x=w292, y=w293) -> (x+y=w289:i32)
                    n274 = Greater?(x=w294, y=w289) -> (0:w295:bool)
                    n275 = case shown="True" w295 {
                      tunnel: w290 -> [_ w303]
                      tunnel: w289 -> [_ w301]
                      tunnel: [w299 w300] -> w288
                      tunnel: w287 -> [_ w300]
                      tunnel: w286 -> [w299 _]
                      frame False {
                      }
                      frame True {
                        n276 = Bundle By Name(cluster=w303, "XStart"=w301) -> (w302:T1)
                        n277 = local write "CCD Area"(w302) -> ()
                      }
                    }
                  }
                }
                n278 = Empty String/Path?(string/path=w261) -> (empty?=w259:bool)
                n279 = case shown="False" w259 {
                  tunnel: [w263 w264] -> w262
                  tunnel: w260 -> [_ w264]
                  tunnel: w261 -> [w263 _]
                  frame False {
                  }
                  frame True {
                  }
                }
                n280 = Empty String/Path?(string/path=w262) -> (empty?=w248:bool)
                n281 = case shown="False" w248 {
                  tunnel: w262 -> [w284 _]
                  frame False {
                    n282 = One Button Dialog(message=w284) -> ()  [unwired: 1 in, 1 out]
                  }
                  frame True {
                  }
                }
              }
            }
          }
          event "Image Mode": Value Change {
            # "For Symphony (II), ADC0 is\n20 kHz and ADC1 is 1 MHz.\nThis couples the selected  ADC\nto the imaging mode selection."
            n283 = event-data() -> ("NewVal"=w307:bool)  [unwired: 1 in, 4 out]
            n284 = Select(t=i8 1, s=w307, f=i8 0) -> (s? t:f=w306:i8)
            n285 = property on="CCD ADC" class="Ring (strict)"("Val(Sgnl)"=w306) -> ()  [unwired: 2 in, 2 out]
          }
          event "CCD Shutter": Value Change {
            n286 = event-data() -> ("NewVal"=w308:bool)  [unwired: 1 in, 4 out]
            n287 = local read "CCD Status"() -> (w309:bool)
            n288 = case shown="False" w309 {
              tunnel: w308 -> [_ w311]
              frame False {
              }
              frame True {
                n289 = local read "JYCCDLib.IJYCCDReqd"() -> (w313:refnum<k7>)
                n290 = local read "CCD Error"() -> (w312:errorcluster)
                n291 = call "Shutter Control.vi"("input error"=w312, "Shutter"=w311, "JYCCDLib.IJYCCDReqd"=w313) -> ("error out"=w314:errorcluster)  [unwired: 1 out]
                n292 = call <vilib>:"Simple Error Handler.vi"("error in (no error)"=w314) -> ("error?"=w310:bool)  [unwired: 4 in, 4 out]
                n293 = local write "CCD Error"(w314) -> ()
                n294 = case shown="True" w310 {
                  tunnel: w311 -> [_ w315]
                  frame False {
                  }
                  frame True {
                    n295 = Not(x=w315) -> (.not. x?=w316:bool)
                    n296 = local write "CCD Shutter"(w316) -> ()
                  }
                }
              }
            }
          }
          event "CCD Acquire": Value Change {
            n297 = event-data() -> ("NewVal"=w317:bool)  [unwired: 1 in, 4 out]
            n298 = case shown="False" w317 {
              frame False {
              }
              frame True {
                n299 = stacked-sequence {
                  frame #0 {
                    n300 = local read "JYCCDLib.IJYCCDReqd"() -> (w318:refnum<k7>)
                    n301 = local read "Image Mode"() -> (w322:bool)
                    n302 = local read "CCD Error"() -> (w319:errorcluster)
                    n303 = control-ref of="CCD Acquire"() -> (w320:refnum<vi>)
                    n304 = control-ref of="CCD Running"() -> (w321:refnum<vi>)
                    n305 = case shown="False" w322 {
                      tunnel: w321 -> [w326 w377]
                      tunnel: w320 -> [w325 w376]
                      tunnel: w319 -> [w324 w378]
                      tunnel: w318 -> [w323 w379]
                      frame False {
                        n306 = local read "CCD Preview"() -> (w327:bool)
                        n307 = local read "Spectrum Settings"() -> (w328:T5)
                        n308 = Unbundle By Name(w328) -> ("Repetitions"=w331:u16)
                        n309 = Select(t=i8 1, s=w327, f=w331) -> (s? t:f=w330:u16)
                        n310 = for {
                          N: w330 -> [w360]
                          tunnel: w323 -> [w352]
                          shift-right: [w365] -> _
                          shift-left: u16[][] [] -> [w366]
                          tunnel: w326 -> [w347]
                          tunnel: w325 -> [w346]
                          tunnel: w324 -> [w345]
                          i -> [w361]
                          stop <- w364 continue-if-true
                          w340 = u16 0 items=["Pixel", "Wavelength", "Energy"] ("Spectrum Axis")
                          w343 = u16 2 items=["Pixel", "Wavelength", "Energy"] ("Spectrum Axis")
                          n311 = Number To Decimal String(number=w360) -> (decimal integer string=w359:string)  [unwired: 1 in]
                          n312 = Increment(x=w361) -> (x+1=w357:i32)
                          n313 = call "Symphony Acquire Spectrum.vi"("Acquire"=w346, "Running"=w347, "Error In"=w345, "ShutterOpen"=TRUE, "JYCCDLib.IJYCCDReqd"=w352) -> ("Acq Time(ms)"=w344:u32, "Raw Data"=w350:i32[][])  [unwired: 5 in]
                          n314 = Number To Decimal String(number=w357) -> (decimal integer string=w358:string)  [unwired: 1 in]
                          n315 = local write "CCD Timing"(w344) -> ()
                          n316 = Index Array(array=w350, index (row)=0) -> (element=w348:i32[])  [unwired: 1 in]
                          n317 = Concatenate Strings(w358, "/" ("string"), w359) -> (w363:string)
                          n318 = local write "CCD Current Rep."(w363) -> ()
                          n319 = Build Array (concatenate)(w348, w366) -> (w365:i32[][])
                          n320 = local read "Wavelengths (nm)"() -> (w338:dbl[])
                          n321 = local read "Spectrum Axis"() -> (w341:u16)
                          n322 = local read "CCD Area"() -> (w337:T1)
                          n323 = call "Symphony Average Spectra.vi"("Repetitions"=w357, "Raw Spectra"=w365) -> ("Raw Spectrum"=w336:dbl[])
                          n324 = Not Equal?(x=w340, y=w341) -> (x != y?=w339:bool)
                          n325 = Equal?(x=w341, y=w343) -> (x = y?=w342:bool)
                          n326 = call "Spectrum Merge Pixels v10.5.0.vi"("CCD Area Format"=w337, "Raw Spectrum"=w336) -> ("Spectrum-Array"=w334:dbl[][])  [unwired: 1 out]
                          n327 = call "Spectrum Merge Wavelengths v10.5.0.vi"("Wavelengths (nm)"=w338, "Raw Spectrum"=w336) -> ("Spectrum-Array"=w333:dbl[][])  [unwired: 1 out]
                          n328 = local read "Spectrum Noise"() -> (w356:i64)
                          n329 = case shown="False" w339 {
                            tunnel: [w367 w368] -> w335
                            tunnel: w333 -> [_ w368]
                            tunnel: w334 -> [w367 _]
                            frame False {
                            }
                            frame True {
                            }
                          }
                          n330 = call "Spectrum Noise Subtraction v10.5.0.vi"("Spectrum Noise"=w356, "Spectrum-Array In"=w335) -> ("Spectrum-Array Out"=w355:dbl[][], "Spectrum-Cluster"=w353:T19)
                          n331 = local write "Spectrum Raw PX"(w334) -> ()
                          n332 = local write "Spectrum Raw WL"(w333) -> ()
                          n333 = case shown="False" w342 {
                            tunnel: w355 -> [_ w371]
                            tunnel: [w369 w370] -> w354
                            tunnel: w353 -> [w369 _]
                            frame False {
                            }
                            frame True {
                              n334 = call "Spectrum Jacobian Transformation v10.5.0.vi"("Spectrum-Array In"=w371) -> ("Spectrum-Cluster"=w370:T19)  [unwired: 1 in, 1 out]
                            }
                          }
                          n335 = local read "CCD Acquire"() -> (w364:bool)
                          n336 = local write "Spectrum"(w354) -> ()
                        }
                      }
                      frame True {
                        n337 = call "Symphony Acquire Image.vi"("Acquire"=w376, "Running"=w377, "Error In"=w378, "ShutterOpen"=TRUE, "JYCCDLib.IJYCCDReqd"=w379) -> ("Acq Time(ms)"=w372:u32, "Raw Data"=w375:i32[][][])  [unwired: 5 in]
                        n338 = local write "CCD Timing"(w372) -> ()
                        n339 = Index Array(array=w375, index (dim 0)=0 ("index (row)")) -> (element=w373:i32[][])  [unwired: 2 in]
                        n340 = local write "Image Raw"(w373) -> ()
                        n341 = local write "Image"(w373) -> ()
                      }
                    }
                  }
                  frame #1 {
                    n342 = local write "CCD Acquire"(FALSE ("Blinkend")) -> ()
                    n343 = local write "CCD Current Rep."("0/0" ("CCD3000 Current Rep.")) -> ()
                    n344 = local read "Spectrum Autosave"() -> (w383:bool)
                    n345 = case shown="False" w383 {
                      frame False {
                      }
                      frame True {
                        n346 = property on="Spectrum Save" class="Bool (strict)"("Val(Sgnl)"=TRUE ("Value (Signaling)")) -> ()  [unwired: 2 in, 2 out]
                      }
                    }
                  }
                }
              }
            }
          }
          event "CCD Preview": Value Change {
            n347 = event-data() -> ("NewVal"=w385:bool)  [unwired: 1 in, 4 out]
            n348 = case shown="False" w385 {
              frame False {
              }
              frame True {
                n349 = property on="CCD Acquire" class="Bool (strict)"("Val(Sgnl)"=TRUE ("Wert (signalisierend)")) -> ()  [unwired: 2 in, 2 out]
              }
            }
          }
          event "ITC Connect": Value Change {
            n350 = event-data() -> ("NewVal"=w387:bool)  [unwired: 1 in, 4 out]
            n351 = stacked-sequence {
              tunnel: w387 -> [_ w389 _]
              frame #0 {
                n352 = property on="ITC Running" class="Bool (strict)"("Blinking"=TRUE ("Blinkend")) -> ()  [unwired: 2 in, 2 out]
              }
              frame #1 {
                n353 = case shown="False" w389 {
                  selector: w389 -> [w394 _]
                  tunnel: [w394 w401] -> w391
                  frame False {
                    # "disconnect"
                    n354 = control-ref of="ITC Running"() -> (w395:refnum<vi>)
                    n355 = property class="Bool (strict)"(reference=w395, "Blinking"=w394, "Value"=w394) -> ()  [unwired: 1 in, 2 out]
                  }
                  frame True {
                    # "connect"
                    n356 = local read "ITC Selector"() -> (w402:u16)
                    n357 = call "ITC503 Connect.vi"("ITC Selector"=w402) -> ("ITC Setup"=w400:T11, "Connected"=w401:bool)
                    n358 = local write "ITC Setup"(w400) -> ()
                    n359 = call "ITC503 Get Values.vi"("ITC Setup"=w400) -> ("ITC503 Current Values"=w399:T2)  [unwired: 1 in, 1 out]
                    n360 = Unbundle By Name(w399) -> ("ITC503 Setpoint"=w396:dbl)
                    n361 = Bundle By Name(cluster=T3 {"ITC503 Set Setpoint"=0.0, "ITC503 Set Auto Heater"=TRUE, "ITC503 Set Auto PID"=TRUE, "P"=0.0, "I"=0.0, "D"=0.0} ("ITC503 Settings"), "ITC503 Set Setpoint"=w396) -> (w397:T3)
                    n362 = local write "ITC Settings"(w397) -> ()
                  }
                }
                n363 = case shown="False" w391 {
                  tunnel: [T15."Disabled and Grayed Out" ("Deaktiviert") T15."Enabled" ("Deaktiviert")] -> w390
                  frame False {
                  }
                  frame True {
                  }
                }
                n364 = local write "ITC Status"(w391) -> ()
                n365 = local write "ITC Connect"(w391) -> ()
                n366 = property on="ITC Configure" class="Bool (strict)"("DisabledEnum"=w390) -> ()  [unwired: 2 in, 2 out]
              }
              frame #2 {
                n367 = property on="ITC Running" class="Bool (strict)"("Blinking"=FALSE ("Blinkend")) -> ()  [unwired: 2 in, 2 out]
                n368 = property on="ITC Read" class="Bool (strict)"("Val(Sgnl)"=TRUE ("Wert (signalisierend)")) -> ()  [unwired: 2 in, 2 out]
              }
            }
          }
          event "ITC Read": Value Change {
            n369 = event-data() -> ("Time"=w406:u32, "NewVal"=w409:bool)  [unwired: 1 in, 3 out]
            n370 = local read "ITC Status"() -> (w408:bool)
            n371 = And(x=w408, y=w409) -> (x .and. y?=w407:bool)
            n372 = case shown="True" w407 {
              tunnel: w406 -> [_ w413]
              tunnel: [u32 0 w412] -> w405
              frame False {
                n373 = property on="ITC Running" class="Bool (strict)"("BoolText.Text"="" ("Boolescher Text.Text")) -> ()  [unwired: 2 in, 2 out]
              }
              frame True {
                n374 = stacked-sequence {
                  seq-local: [_ w419 _ _] -> [_ _ w440 _]
                  seq-local: [w414 _ _ _] -> [_ _ _ w448]
                  tunnel: w413 -> [_ w420 _ _]
                  tunnel: [_ _ _ w449] -> w412
                  frame #0 {
                    n375 = Tick Count (ms)() -> (millisecond timer value=w414:u32)
                  }
                  frame #1 {
                    n376 = local read "ITC Setup"() -> (w425:T11)
                    n377 = local read "ITC Gradient Time"() -> (w424:i64)
                    n378 = call "ITC503 Get Values.vi"("ITC Setup"=w425) -> ("ITC503 Current Values"=w419:T2)  [unwired: 1 in, 1 out]
                    n379 = local read "ITC Temp Storage"() -> (w418:dbl)
                    n380 = Unbundle By Name(w419) -> ("ITC503 Temperature"=w417:dbl)
                    n381 = Subtract(x=w420, y=w424) -> (x-y=w423:i64)
                    n382 = Divide(x=w423, y=i64 1000) -> (x/y=w421:dbl)
                    n383 = Equal To 0?(x=w417) -> (x = 0?=w416:bool)
                    n384 = case shown="False" w416 {
                      tunnel: w421 -> [w431 _]
                      tunnel: w419 -> [w430 _]
                      tunnel: w418 -> [w429 _]
                      tunnel: w417 -> [w427 _]
                      frame False {
                        n385 = Subtract(x=w427, y=w429) -> (x-y=w428:dbl)
                        n386 = Divide(x=w428, y=w431) -> (x/y=w432:dbl)
                        n387 = Bundle By Name(cluster=w430, "ITC503 Gradient"=w432) -> (w426:T2)
                        n388 = local write "ITC Current Values"(w426) -> ()
                        n389 = global write "Global Variables.vi" "Global ITC Values"(w426) -> ()
                      }
                      frame True {
                      }
                    }
                    n390 = Not(x=w416) -> (.not. x?=w415:bool)
                    n391 = local write "ITC Status"(w415) -> ()
                  }
                  frame #2 {
                    n392 = Unbundle By Name(w440) -> ("ITC503 Temperature"=w435:dbl, "ITC503 Setpoint"=w441:dbl)
                    n393 = Subtract(x=w435, y=w441) -> (x-y=w442:dbl)
                    n394 = Number To Fractional String(number=w435, precision (6)=i16 2 ("Genauigkeit (6)")) -> (F-format string=w438:string)  [unwired: 2 in]
                    n395 = local write "ITC Temp Storage"(w435) -> ()
                    n396 = Absolute Value(x=w442) -> (abs(x)=w443:dbl)
                    n397 = String Subset(string=w438, length (rest)=5 ("Länge (Rest)")) -> (substring=w436:string)  [unwired: 1 in]
                    n398 = Less?(x=w443, y=2.0) -> (x < y?=w434:bool)
                    n399 = case shown="True" w434 {
                      tunnel: [u32 16711680 u32 0] -> w433
                      frame False {
                      }
                      frame True {
                      }
                    }
                    n400 = property on="ITC Running" class="Bool (strict)"("Value"=w434, "BoolText.Text"=w436, "BoolText.TextColor"=w433) -> ()  [unwired: 2 in, 2 out]
                  }
                  frame #3 {
                    n401 = Tick Count (ms)() -> (millisecond timer value=w447:u32)
                    n402 = local write "ITC Gradient Time"(w447) -> ()
                    n403 = Subtract(x=w447, y=w448) -> (x-y=w449:u32)
                  }
                }
              }
            }
            n404 = local write "ITC Timing"(w405) -> ()
          }
          event "ITC Configure": Value Change {
            n405 = event-data() -> ("NewVal"=w450:bool)  [unwired: 1 in, 4 out]
            n406 = stacked-sequence {
              tunnel: w450 -> [_ w452 _]
              frame #0 {
                n407 = property on="ITC Running" class="Bool (strict)"("Blinking"=TRUE ("Blinkend")) -> ()  [unwired: 2 in, 2 out]
              }
              frame #1 {
                n408 = local read "ITC Status"() -> (w454:bool)
                n409 = And(x=w454, y=w452) -> (x .and. y?=w453:bool)
                n410 = case shown="True" w453 {
                  frame False {
                  }
                  frame True {
                    n411 = local read "ITC Settings"() -> (w455:T3)
                    n412 = local read "ITC Setup"() -> (w456:T11)
                    n413 = call "ITC503 Set Values.vi"("Set Channel"=i16 1, "ITC503 Settings"=w455, "ITC Setup"=w456) -> ()  [unwired: 2 in]
                  }
                }
              }
              frame #2 {
                w459 = FALSE ("Blinkend")
                n414 = property on="ITC Running" class="Bool (strict)"("Blinking"=w459) -> ()  [unwired: 2 in, 2 out]
                n415 = local write "ITC Configure"(w459) -> ()
                n416 = property on="ITC Read" class="Bool (strict)"("Val(Sgnl)"=TRUE ("Wert (signalisierend)")) -> ()  [unwired: 2 in, 2 out]
              }
            }
          }
          event "Drive Connect": Value Change {
            n417 = event-data() -> ("NewVal"=w460:bool)  [unwired: 1 in, 4 out]
            n418 = stacked-sequence {
              tunnel: w460 -> [_ w463 _ _]
              frame #0 {
                n419 = property on="Drive Running" class="Bool (strict)"("Blinking"=TRUE ("Blinkend")) -> ()  [unwired: 2 in, 2 out]
              }
              frame #1 {
                n420 = local read "Drive Connection"() -> (w464:refnum<visa-resource-name>)
                n421 = case shown="False" w463 {
                  tunnel: w464 -> [w469 w471]
                  tunnel: [TRUE ("Success") w470] -> w462
                  frame False {
                    n422 = call "NPC3SG Close.vi"("Drive Visa Name"=w469) -> ()  [unwired: 4 in]
                  }
                  frame True {
                    n423 = call "NPC3SG Connect v10.6.1.vi"("Drive Port"=w471) -> ("Success"=w470:bool)  [unwired: 2 in, 1 out]
                  }
                }
                n424 = Not(x=w463) -> (.not. x?=w466:bool)
                n425 = Exclusive Or(1:w466, 2:w462) -> (0:w467:bool)
                n426 = local write "Drive Connect"(w467) -> ()
                n427 = local write "Drive Status"(w467) -> ()
                n428 = case shown="False" w467 {
                  tunnel: [T15."Disabled and Grayed Out" ("Deaktiviert") T15."Enabled" ("Deaktiviert")] -> w465
                  frame False {
                  }
                  frame True {
                  }
                }
                n429 = property on="Drive Live Controls" class="Clust (strict)"("DisabledEnum"=w465) -> ()  [unwired: 2 in, 2 out]
                n430 = property on="Drive GoTo" class="Bool (strict)"("DisabledEnum"=w465) -> ()  [unwired: 2 in, 2 out]
              }
              frame #2 {
                # "prepare mirroring values to target controls"
                n431 = local write "Drive Copy Target"(TRUE ("Copy Drive Target")) -> ()
              }
              frame #3 {
                n432 = property on="Drive Running" class="Bool (strict)"("Blinking"=FALSE ("Blinkend")) -> ()  [unwired: 2 in, 2 out]
                n433 = property on="Drive Read" class="Bool (strict)"("Val(Sgnl)"=TRUE ("Wert (signalisierend)")) -> ()  [unwired: 2 in, 2 out]
              }
            }
          }
          event "Drive Read": Value Change {
            n434 = event-data() -> ("NewVal"=w480:bool)  [unwired: 1 in, 4 out]
            n435 = local read "Drive Status"() -> (w479:bool)
            n436 = And(x=w479, y=w480) -> (x .and. y?=w478:bool)
            n437 = case shown="True" w478 {
              tunnel: [u32 0 w482] -> w477
              frame False {
              }
              frame True {
                n438 = stacked-sequence {
                  seq-local: [w483 _ _ _] -> [_ _ _ w489]
                  tunnel: [_ _ _ w488] -> w482
                  frame #0 {
                    n439 = Tick Count (ms)() -> (millisecond timer value=w483:u32)
                  }
                  frame #1 {
                    n440 = local read "Drive Connection"() -> (w485:refnum<visa-resource-name>)
                    n441 = call "NPC3SG Get Positions v10.6.1.vi"("Drive Visa Name"=w485) -> ("Drive Current Values"=w484:T4)  [unwired: 6 in]
                    n442 = local write "Drive Live Current Values"(w484) -> ()
                    n443 = local write "Drive Current Values"(w484) -> ()
                    n444 = global write "Global Variables.vi" "Global Piezo Position"(w484) -> ()
                  }
                  frame #2 {
                    n445 = local read "Drive Copy Target"() -> (w486:bool)
                    n446 = case shown="True" w486 {
                      frame False {
                      }
                      frame True {
                        n447 = property on="Drive Copy Target" class="Bool (strict)"("Val(Sgnl)"=TRUE ("Value (Signaling)")) -> ()  [unwired: 2 in, 2 out]
                      }
                    }
                  }
                  frame #3 {
                    n448 = Tick Count (ms)() -> (millisecond timer value=w490:u32)
                    n449 = Subtract(x=w490, y=w489) -> (x-y=w488:u32)
                  }
                }
              }
            }
            "Drive Timing" <- w477
          }
          event "Drive GoTo": Value Change {
            n450 = event-data() -> ("NewVal"=w491:bool)  [unwired: 1 in, 4 out]
            n451 = stacked-sequence {
              tunnel: w491 -> [_ w493 _]
              frame #0 {
                n452 = property on="Drive Running" class="Bool (strict)"("Blinking"=TRUE ("Blinkend")) -> ()  [unwired: 2 in, 2 out]
              }
              frame #1 {
                n453 = local read "Drive Status"() -> (w495:bool)
                n454 = And(x=w495, y=w493) -> (x .and. y?=w494:bool)
                n455 = case shown="True" w494 {
                  frame False {
                  }
                  frame True {
                    n456 = local read "Drive New Positions"() -> (w497:T6)
                    n457 = local read "Drive Connection"() -> (w496:refnum<visa-resource-name>)
                    n458 = control-ref of="Drive Running"() -> (w498:refnum<vi>)
                    n459 = call "NPC3SG Move Absolute v10.6.1.vi"("Running"=w498, "Drive New Abs. Positions"=w497, "Drive Visa Name"=w496) -> ()  [unwired: 2 in]
                  }
                }
              }
              frame #2 {
                w500 = FALSE ("Blinkend")
                n460 = local write "Drive GoTo"(w500) -> ()
                n461 = property on="Drive Running" class="Bool (strict)"("Blinking"=w500) -> ()  [unwired: 2 in, 2 out]
                n462 = property on="Drive Read" class="Bool (strict)"("Val(Sgnl)"=TRUE ("Wert (signalisierend)")) -> ()  [unwired: 2 in, 2 out]
              }
            }
          }
          event Value Change {
            n463 = event-data() -> ("NewVal"=w502:bool)  [unwired: 1 in, 4 out]
            n464 = local read "Drive Status"() -> (w503:bool)
            n465 = And(x=w503, y=w502) -> (x .and. y?=w501:bool)
            n466 = case shown="True" w501 {
              frame False {
              }
              frame True {
                n467 = stacked-sequence {
                  seq-local: [w504 _ _] -> [_ _ _]
                  frame #0 {
                    # "Move and Read"
                    n468 = flat-sequence {
                      tunnel: [w511] -> w507
                      tunnel: [w509] -> w506
                      tunnel: w507 -> [w513]
                      tunnel: w506 -> [w514]
                      tunnel: [w512] -> w505
                      tunnel: w505 -> [w519]
                      tunnel: [w519] -> w504
                      frame #0 {
                        n469 = local read "Drive Live Controls"() -> (w509:T7)
                        n470 = local read "Drive Connection"() -> (w508:refnum<visa-resource-name>)
                        n471 = control-ref of="Drive Running"() -> (w510:refnum<vi>)
                        n472 = call "NPC3SG Live Control v10.6.1.vi"("Running"=w510, "Drive Live Controls"=w509, "Drive Visa Name"=w508) -> ("Reset Switches"=w511:bool)  [unwired: 1 in]
                      }
                      frame #1 {
                        n473 = case shown="False" w513 {
                          tunnel: w514 -> [w515 w518]
                          tunnel: [w515 w517] -> w512
                          frame False {
                          }
                          frame True {
                            w516 = FALSE ("Move Out")
                            n474 = Bundle By Name(cluster=w518, "Move Home"=w516, "Move Down"=w516, "Move Up"=w516, "Move Left"=w516, "Move Right"=w516, "Move Out"=w516, "Move In"=w516) -> (w517:T7)
                          }
                        }
                      }
                      frame #2 {
                        n475 = local write "Drive Live Controls"(w519) -> ()
                      }
                    }
                  }
                  frame #1 {
                    n476 = local write "Drive Copy Target"(TRUE ("Copy Drive Target")) -> ()
                  }
                  frame #2 {
                    n477 = property on="Drive Read" class="Bool (strict)"("Val(Sgnl)"=TRUE ("Wert (signalisierend)")) -> ()  [unwired: 2 in, 2 out]
                  }
                }
              }
            }
          }
          event "Drive Copy Target": Value Change {
            # "this event is triggered after drive readout\nit should usually not be triggered directly by signaling"
            n478 = event-data() -> ("NewVal"=w522:bool)  [unwired: 1 in, 4 out]
            n479 = case shown="True" w522 {
              frame False {
              }
              frame True {
                n480 = stacked-sequence {
                  frame #0 {
                    n481 = local read "Drive Current Values"() -> (w523:T4)
                    n482 = local write "Drive New Positions"(w523) -> ()
                  }
                  frame #1 {
                    n483 = local write "Drive Copy Target"(FALSE ("Copy Drive Target")) -> ()
                  }
                }
              }
            }
          }
          event "Wavelength Recalculate": Value Change {
            n484 = event-data() -> ("NewVal"=w525:bool)  [unwired: 1 in, 4 out]
            n485 = case shown="False" w525 {
              frame False {
              }
              frame True {
                n486 = local read "Mono Current Values"() -> (w528:T9)
                n487 = local read "CCD Area"() -> (w526:T1)
                n488 = call "iHR550 Convert Axis v10.5.0.vi"("CCD Area Format"=w526, "iHR Current Values"=w528) -> ("Wavelengths (nm)"=w527:dbl[])
                n489 = local write "Wavelengths (nm)"(w527) -> ()
                n490 = global write "Global Variables.vi" "Global Wavelengths (nm)"(w527) -> ()
              }
            }
          }
          event Value Change {
            n491 = event-data() -> ("NewVal"=w530:dbl)  [unwired: 1 in, 4 out]
            n492 = local read "JYCCDLib.IJYCCDReqd"() -> (w529:refnum<k7>)
            n493 = call "Symphony Set Integration Time.vi"("JYCCDLib.IJYCCDReqd"=w529, "Integration (s)"=w530) -> ()  [unwired: 13 in, 1 out]
          }
          event "Spectrum Axis": Value Change {
            w543 = u16 2 items=["Pixel", "Wavelength", "Energy"] ("Spectrum Axis")
            w545 = u16 0 items=["Pixel", "Wavelength", "Energy"] ("Spectrum Axis")
            n494 = event-data() -> ("NewVal"=w541:u16)  [unwired: 1 in, 4 out]
            n495 = Equal?(x=w541, y=w545) -> (x = y?=w544:bool)
            n496 = case shown="True" w544 {
              tunnel: [w563 w565] -> w542
              tunnel: [w562 w564] -> w537
              tunnel: "Pixel" ("X Scale.Name Label.Text") -> [_ w564]
              tunnel: "Wavelength (nm)" ("X Scale.Name Label.Text") -> [w562 _]
              frame False {
                n497 = local read "Spectrum Raw WL"() -> (w563:dbl[][])
              }
              frame True {
                n498 = local read "Spectrum Raw PX"() -> (w565:dbl[][])
              }
            }
            n499 = local read "Spectrum Noise"() -> (w532:i64)
            n500 = Equal?(x=w541, y=w543) -> (x = y?=w540:bool)
            n501 = call "Spectrum Noise Subtraction v10.5.0.vi"("Spectrum Noise"=w532, "Spectrum-Array In"=w542) -> ("Spectrum-Array Out"=w539:dbl[][], "Spectrum-Cluster"=w531:T19)
            n502 = case shown="True" w540 {
              tunnel: w539 -> [_ w553]
              tunnel: [w547 w552] -> w538
              tunnel: w531 -> [w547 w551]
              tunnel: w537 -> [w546 w548]
              tunnel: [w546 w550] -> w534
              tunnel: "Energy (eV)" ("X Scale.Name Label.Text") -> [_ w549]
              tunnel: w532 -> [_ w554]
              frame False {
              }
              frame True {
                # "Jacobian Transformation requires noise subtraction"
                n503 = Greater Than 0?(x=w554) -> (x > 0?=w555:bool)
                n504 = case shown="False" w555 {
                  tunnel: w553 -> [_ w561]
                  tunnel: [w557 w560] -> w552
                  tunnel: w551 -> [w557 _]
                  tunnel: [w556 w559] -> w550
                  tunnel: w549 -> [_ w559]
                  tunnel: w548 -> [w556 _]
                  frame False {
                    w558 = u16 1 items=["Pixel", "Wavelength", "Energy"] ("Spectrum Axis")
                    n505 = call "Display Message to User"() -> ()  [unwired: 10 in, 2 out]
                    n506 = local write "Spectrum Axis"(w558) -> ()
                  }
                  frame True {
                    n507 = call "Spectrum Jacobian Transformation v10.5.0.vi"("Spectrum-Array In"=w561) -> ("Spectrum-Cluster"=w560:T19)  [unwired: 1 in, 1 out]
                  }
                }
              }
            }
            n508 = local write "Spectrum"(w538) -> ()
            n509 = property on="Spectrum" class="XYGraph (strict)"("XScale.NameLbl.Text"=w534) -> ()  [unwired: 2 in, 2 out]
          }
          event "Spectrum Noise": Value Change {
            n510 = event-data() -> ("NewVal"=w568:i64)  [unwired: 1 in, 4 out]
            n511 = Greater Than 0?(x=w568) -> (x > 0?=w567:bool)
            n512 = case shown="False" w567 {
              tunnel: [w569 w570] -> w566
              frame False {
                w569 = u16 1 items=["Pixel", "Wavelength", "Energy"] ("Spectrum Axis")
                # "Disable Jacobian Transformation"
              }
              frame True {
                n513 = local read "Spectrum Axis"() -> (w570:u16)
              }
            }
            n514 = property on="Spectrum Axis" class="Ring (strict)"("Val(Sgnl)"=w566) -> ()  [unwired: 2 in, 2 out]
          }
          event "Spectrum Save": Value Change {
            n515 = event-data() -> ("NewVal"=w571:bool)  [unwired: 1 in, 4 out]
            n516 = stacked-sequence {
              tunnel: w571 -> [w572 _]
              frame #0 {
                n517 = case shown="True" w572 {
                  frame False {
                  }
                  frame True {
                    n518 = local read "Mono Current Values"() -> (w575:T9)
                    n519 = local read "Drive Current Values"() -> (w573:T4)
                    n520 = local read "ITC Current Values"() -> (w576:T2)
                    n521 = local read "Spectrum Settings"() -> (w574:T5)
                    n522 = local read "CCD Temperature"() -> (w581:dbl)
                    n523 = local read "CCD Area"() -> (w578:T1)
                    n524 = local read "CCD ADC"() -> (w580:u16)
                    n525 = local read "CCD Gain"() -> (w579:u16)
                    n526 = local read "Image Mode"() -> (w587:bool)
                    n527 = call "Export_fileName v10.6.0.vi"("ITC503 Current Values"=w576, "iHR Current Values"=w575, "Spectra Settings"=w574, "Drive Current Values"=w573) -> ("Filename"=w577:string)  [unwired: 1 in]
                    n528 = case shown="True" w587 {
                      tunnel: [w588 w592] -> w585
                      tunnel: ["Spectrum" ("Export Type") "Image" ("Export Type")] -> w584
                      tunnel: [w589 w596] -> w582
                      tunnel: w578 -> [_ w591]
                      tunnel: w577 -> [w588 w594]
                      frame False {
                        n529 = local read "Spectrum Raw WL"() -> (w589:dbl[][])
                      }
                      frame True {
                        n530 = local read "Image Raw"() -> (w595:i32[][])
                        n531 = Concatenate Strings(w594, "_img" ("string")) -> (w592:string)
                        n532 = call "Image Merge Axes v10.5.1.vi"("Image In"=w595, "CCD Area Format"=w591) -> ("Image Out"=w596:dbl[][])  [unwired: 13 in]
                      }
                    }
                    n533 = local read "Spectrum Autosave"() -> (w583:bool)
                    n534 = local read "Auto Folder"() -> (w586:path)
                    n535 = call "Export_2DtoTxt v10.6.0.vi"("ITC503 Current Values"=w576, "iHR Current Values"=w575, "CCD Temperature"=w581, "CCD Area"=w578, "CCD ADC"=w580, "CCD Gain"=w579, "Auto?"=w583, "Export Type"=w584, "Spectra Settings"=w574, "Filename"=w585, "Data (2D)"=w582, "Auto Folder"=w586) -> ()  [unwired: 7 in, 1 out]
                  }
                }
              }
              frame #1 {
                n536 = local write "Spectrum Save"(FALSE ("Spectrum Save")) -> ()
              }
            }
          }
          event "Spectrum Load": Value Change {
            n537 = event-data() -> ("NewVal"=w599:bool)  [unwired: 1 in, 4 out]
            n538 = case shown="True" w599 {
              frame False {
              }
              frame True {
                n539 = stacked-sequence {
                  seq-local: [w600 _ _] -> [_ w603 _]
                  frame #0 {
                    n540 = call "Load Spectrum.vi"() -> ("Intensity"=w600:dbl[], "Wavelength"=w602:dbl[])  [unwired: 3 in, 1 out]
                    n541 = Build Array(w602, w600) -> (w601:dbl[][])
                    n542 = local write "Spectrum Raw WL"(w601) -> ()
                  }
                  frame #1 {
                    n543 = call <vilib>:"Median.vi"("X"=w603) -> ("median"=w605:dbl)  [unwired: 1 out]
                    n544 = To Long Integer(number=w605) -> (32bit integer=w604:i32)
                    n545 = property on="Spectrum Noise" class="DigNum (strict)"("Val(Sgnl)"=w604) -> ()  [unwired: 2 in, 2 out]
                  }
                  frame #2 {
                    n546 = local write "Spectrum Load"(FALSE ("Spectrum Load")) -> ()
                  }
                }
              }
            }
          }
          event "Spectrum Autosave": Value Change {
            n547 = event-data() -> ("NewVal"=w608:bool)  [unwired: 1 in, 4 out]
            n548 = case shown="False" w608 {
              tunnel: [path "" w614] -> w607
              frame False {
              }
              frame True {
                n549 = call "File Dialog"("prompt"="Choose Save Folder") -> ("selected path"=w616:path, "cancelled"=w610:bool, "error out"=w612:errorcluster)  [unwired: 11 in, 1 out]
                n550 = call <vilib>:"Simple Error Handler.vi"("error in (no error)"=w612) -> ("error?"=w611:bool)  [unwired: 4 in, 4 out]
                n551 = Or(x=w610, y=w611) -> (x .or. y?=w613:bool)
                n552 = case shown="True" w613 {
                  tunnel: w616 -> [w617 _]
                  tunnel: [w617 path ""] -> w614
                  frame False {
                  }
                  frame True {
                    n553 = local write "Spectrum Autosave"(FALSE ("Spectrum Autosave")) -> ()
                  }
                }
              }
            }
            n554 = local write "Auto Folder"(w607) -> ()
          }
          event "Spectrum Maximize": Value Change {
            # "Currently disabled by hiding control!"
            n555 = event-data() -> ("NewVal"=w620:bool)  [unwired: 1 in, 4 out]
            n556 = case shown="False" w620 {
              frame False {
                n557 = local read "Spectrum Properties"() -> (w623:cluster{"Position":T10, "Plot Area Size":T10})
                n558 = Unbundle(w623) -> ("Position"=w622:T10, "Plot Area Size"=w621:T10)
                n559 = stacked-sequence {
                  tunnel: w622 -> [_ w625]
                  tunnel: w621 -> [w624 _]
                  frame #0 {
                    n560 = property on="Spectrum" class="XYGraph (strict)"("Plot Area Size"=w624) -> ()  [unwired: 2 in, 2 out]
                  }
                  frame #1 {
                    n561 = property on="Spectrum" class="XYGraph (strict)"("Position"=w625) -> ()  [unwired: 2 in, 2 out]
                  }
                }
              }
              frame True {
                n562 = property on="Spectrum" class="XYGraph (strict)"() -> ("Bounds"=w646:T10, "Plot Area Size"=w645:T10, "Position"=w643:T20)  [unwired: 2 in, 2 out]
                n563 = Bundle("Position"=w643, "Plot Area Size"=w645) -> (w644:cluster{"Position":T20, "Plot Area Size":T10})  [unwired: 1 in]
                n564 = Unbundle By Name(w646) -> ("Width"=w650:u32, "Height"=w651:u32)
                n565 = Unbundle By Name(w645) -> ("Width"=w653:u32, "Height"=w652:u32)
                n566 = property on="Register" class="TabCtl (strict)"() -> ("Bounds"=w649:T10, "Position"=w638:T20, "Width"=w629:u32, "Height"=w628:u32)  [unwired: 2 in, 2 out]
                n567 = local write "Spectrum Properties"(w644) -> ()
                n568 = Subtract(x=w650, y=w653) -> (x-y=w642:u32)
                n569 = Subtract(x=w651, y=w652) -> (x-y=w639:u32)
                n570 = Add(x=w642, y=u32 25) -> (x+y=w641:u32)
                n571 = Add(x=w639, y=u32 70) -> (x+y=w640:u32)
                n572 = Subtract(x=w629, y=w641) -> (x-y=w648:u32)
                n573 = Subtract(x=w628, y=w640) -> (x-y=w647:u32)
                n574 = Bundle By Name(cluster=w649, "Width"=w648, "Height"=w647) -> (w626:T10)
                n575 = Unbundle By Name(w638) -> ("Left"=w637:i32, "Top"=w634:i32)
                n576 = Add(x=w637, y=20) -> (x+y=w636:i32)
                n577 = Add(x=w634, y=50) -> (x+y=w635:i32)
                n578 = Bundle By Name(cluster=w638, "Left"=w636, "Top"=w635) -> (w627:T20)
                n579 = stacked-sequence {
                  tunnel: w627 -> [w654 _]
                  tunnel: w626 -> [_ w655]
                  frame #0 {
                    n580 = property on="Spectrum" class="XYGraph (strict)"("Position"=w654) -> ()  [unwired: 2 in, 2 out]
                  }
                  frame #1 {
                    n581 = property on="Spectrum" class="XYGraph (strict)"("Plot Area Size"=w655) -> ()  [unwired: 2 in, 2 out]
                  }
                }
              }
            }
          }
          event "Mapping Start": Value Change {
            n582 = event-data() -> ("NewVal"=w656:bool)  [unwired: 1 in, 4 out]
            n583 = case shown="True" w656 {
              frame False {
              }
              frame True {
                n584 = stacked-sequence {
                  frame #0 {
                    # "Make sure we do not try mapping in the image mode."
                    n585 = flat-sequence {
                      frame #0 {
                        n586 = property on="Image Mode" class="Bool (strict)"("Val(Sgnl)"=FALSE ("Value (Signaling)")) -> ()  [unwired: 2 in, 2 out]
                      }
                      frame #1 {
                        n587 = property on="CCD Configure" class="Bool (strict)"("Val(Sgnl)"=TRUE ("Value (Signaling)")) -> ()  [unwired: 2 in, 2 out]
                      }
                    }
                  }
                  frame #1 {
                    n588 = local read "JYCCDLib.IJYCCDReqd"() -> (w697:refnum<k7>)
                    n589 = local read "Drive Current Values"() -> (w692:T4)
                    n590 = local read "ITC Current Values"() -> (w694:T2)
                    n591 = local read "Mono Current Values"() -> (w693:T9)
                    n592 = local read "CCD Temperature"() -> (w699:dbl)
                    n593 = vi-ref "Mapping v10.6.1.vi"() -> (w680:refnum<vi>)
                    n594 = local read "Wavelengths (nm)"() -> (w695:dbl[])
                    n595 = local read "Drive Status"() -> (w691:bool)
                    n596 = local read "Drive Connection"() -> (w696:refnum<visa-resource-name>)
                    n597 = local read "Spectrum Settings"() -> (w698:T5)
                    n598 = local read "CCD Status"() -> (w689:bool)
                    n599 = local read "CCD ADC"() -> (w660:u16)
                    n600 = local read "CCD Area"() -> (w662:T1)
                    n601 = local read "CCD Gain"() -> (w661:u16)
                    n602 = local read "CCD Status"() -> (w673:bool)
                    n603 = Not(x=w691) -> (.not. x?=w690:bool)
                    n604 = Not(x=w689) -> (.not. x?=w688:bool)
                    n605 = Not(x=w673) -> (.not. x?=w672:bool)
                    n606 = Bundle By Name(cluster=T18 {"Drive Connection Port"="", "ITC503 Current Values"={"ITC503 Heater"=0.0, "ITC503 Temperature"=0.0, "ITC503 P"=0.0, "ITC503 I"=0.0, "ITC503 D"=0.0, "ITC503 Setpoint"=0.0, "ITC503 Gradient"=0.0, "ITC503 Heater Auto"=FALSE, "ITC503 PID Auto"=FALSE}, "Wavelengths (nm)"=[], "Drive Current Values"={"Drive X Position"=0.0, "Drive Y Position"=0.0, "Drive Z Position"=0.0}, "iHR Current Values"={"iHR 550 Front Entrance"=0.0, "iHR550 Side Exit"=0.0, "iHR550 Wavelength"=897.9988, "iHR550 Exit Mirror"=2, "iHR550 Grating"="1", "Grating Index"=1}, "Spectra Settings"={"Integration Time"=1.0, "Repetitions"=1, "Mapping Spectra"=TRUE}, "CCD3500 Temperature"=0.0, "Simulate Drive"=FALSE, "Simulate Spectra"=FALSE, "JYCCDLib.IJYCCDReqd"=refnum, "CCD Area"={"XStart"=1, "YStart"=1, "XStop"=2048, "YStop"=512, "XBin"=1, "YBin"=1}, "CCD Gain"=1, "CCD ADC"=0} ("Input Parameters"), "JYCCDLib.IJYCCDReqd"=w697, "Drive Connection Port"=w696, "ITC503 Current Values"=w694, "Wavelengths (nm)"=w695, "Drive Current Values"=w692, "iHR Current Values"=w693, "Spectra Settings"=w698, "CCD3500 Temperature"=w699, "Simulate Drive"=w690, "Simulate Spectra"=w688, "CCD Area"=w662, "CCD Gain"=w661, "CCD ADC"=w660) -> (w681:T18)
                    n607 = invoke class="VI" method="Ctrl Val.Set"(reference=w680, "Control Name"="Simulate Spectra", "Value"=w672) -> (reference out=w679:refnum<vi>, error out=w674:errorcluster)  [unwired: 2 in, 3 out]
                    n608 = local read "Drive Status"() -> (w671:bool)
                    n609 = Not(x=w671) -> (.not. x?=w670:bool)
                    n610 = invoke class="VI" method="Ctrl Val.Set"(reference=w679, error in=w674, "Control Name"="Simulate Drive", "Value"=w670) -> (reference out=w678:refnum<vi>, error out=w675:errorcluster)  [unwired: 1 in, 3 out]
                    n611 = invoke class="VI" method="Ctrl Val.Set"(reference=w678, error in=w675, "Control Name"="Input Parameters", "Value"=w681) -> (reference out=w668:refnum<vi>, error out=w665:errorcluster)  [unwired: 1 in, 3 out]
                    n612 = property on="Measurement Running" class="Bool (strict)"("Blinking"=TRUE ("Blinkend")) -> ()  [unwired: 2 in, 2 out]
                    n613 = invoke class="VI" method="Ctrl Val.Set"(reference=w668, error in=w665, "Control Name"="AutoClose", "Value"=TRUE ("Blinkend")) -> (reference out=w667:refnum<vi>, error out=w666:errorcluster)  [unwired: 1 in, 3 out]
                    n614 = invoke on="Invoke Node" class="VI" method="FP.Open"(reference=w667, error in=w666, "Activate"=TRUE ("Activate?")) -> (reference out=w683:refnum<vi>, error out=w682:errorcluster)  [unwired: 2 in, 3 out]
                    n615 = invoke on="Invoke Node" class="VI" method="Run VI"(reference=w683, error in=w682, "Wait until done"=FALSE ("Wait Until Done"), "Auto Dispose Ref"=TRUE ("Auto Dispose Reference")) -> ()  [unwired: 1 in, 5 out]
                  }
                }
              }
            }
          }
          event "Video Show": Value Change {
            n616 = event-data() -> ("NewVal"=w700:bool)  [unwired: 1 in, 4 out]
            n617 = case shown="True" w700 {
              frame False {
                n618 = call "Video Toolset Stop.vi"() -> ()  [unwired: 3 in]
              }
              frame True {
                n619 = local read "Snapshot Folder"() -> (w702:path)
                n620 = local read "Camera Name"() -> (w701:string)
                n621 = call "Video Toolset Start.vi"("Snapshot Folder"=w702, "Camera Name"=w701) -> ()  [unwired: 1 in]
              }
            }
          }
        }
      }
    }
    frame #3 {
      # "Close Connections"
      n622 = control-ref of="Dieses VI"() -> (w703:refnum<vi>)
      n623 = invoke class="VI" method="Default Vals.Reinit All"(reference=w703) -> ()  [unwired: 2 in, 3 out]
    }
  }
